vi "main_2CAN.vi"() -> ()   [LabVIEW 2021]
uses:
  <vilib>/xnet/xnet.llb/XNET Frame CAN.ctl
  <vilib>/xnet/xnet.llb/XNET Frame Type CAN.ctl
  Helper functions/General Purpose/measurements.ctl
  Helper functions/General Purpose/measurements_SC.ctl
  Helper functions/Time-sync/time_sync/TypeDef/Synch_shift--cluster.ctl
  <vilib>/Platform/TimedLoop/XDataNode/timing_clust.ctl
  <vilib>/Platform/TimedLoop/XDataNode/nitl_modes.ctl
  <vilib>/Platform/TimedLoop/XDataNode/wakeup.ctl
  Helper functions/communication/PVemulator_Central.ctl
  Helper functions/communication/PVemulator_Central_Info.ctl
  Helper functions/communication/PVemulator_Central_Data.ctl
  Helper functions/communication/SC_references.ctl
  Helper functions/central data acquisition/MeteoBoxCentral.ctl
  Helper functions/central data acquisition/MeteoBoxCentral_Info.ctl
  Helper functions/central data acquisition/MeteoBoxCentral_Data.ctl
  <vilib>/Analysis/baseanly.llb/Mean (DBL).vi
  <vilib>/xnet/xnet.llb/XNET Write (Frame CAN).vi
  <vilib>/xnet/xnet.llb/XNET Read (Frame CAN).vi
  <vilib>/Platform/TimedLoop/XDataNode/XDataNode.xnode
  <vilib>/Platform/TimedLoop/XDataNode/XDNodeRunTimeDep.lvlib
  <userlib>/_OpenG.lib/boolean/boolean.llb/openg_boolean__ogtk.lvlib
  <vilib>/Analysis/NI_AALBase.lvlib
panel:
  out "Finished Late? [i-1]":bool
  out "Iteration Duration":i64
  out "SOC_plot":cluster{"SOC":dbl, "mean":dbl}(graph)
  in  "Vdc_bias":dbl=-4.0 format="%#_13g"
  out "CAN OUT 2":T1 {"payload" format="%x"; "timestamp" format="%<%.7X\n%x>T"; "type" items=["CAN Data"=0, "CAN Remote"=1, "CAN Bus Error"=2, "CAN 2.0 Data"=8, "CAN FD Data"=16, "CAN FD+BRS Data"=24, "J1939 Data"=192, "Delay"=224, "Log Trigger"=225, "Start Trigger"=226]; "identifier" format="%x"}
  out "CAN frame":T1 {"payload" format="%x"; "timestamp" format="%<%.7X\n%x>T"; "type" items=["CAN Data"=0, "CAN Remote"=1, "CAN Bus Error"=2, "CAN 2.0 Data"=8, "CAN FD Data"=16, "CAN FD+BRS Data"=24, "J1939 Data"=192, "Delay"=224, "Log Trigger"=225, "Start Trigger"=226]; "identifier" format="%x"}
  out "Period":i64
  out "time_sc":timestamp
  out "start following SC pre":bool
  out "forming?":bool
  out "Ready SC":bool
  out "OFF SC":bool
  out "V slider 31":dbl(slide) caption="V-i" max=-10.0 scale=0.0..100.0 scale format="%#_4g"
  in  "SEND sp SC":bool
  in  "Start following SC":bool
  in  "Start forming SC":bool
  in  "Vdc SC":dbl=720.0
  out "Synch Monitor":string[][](table)
  in  "Loop Time":u32=125
  out "Error out":errorcluster
  in  "Timeout [ms]":i32=3000
  out "Offset from TR (ns)":dbl
  out "Status Out":T3
  out "ON SC":bool
  out "state SC":u16
  out "measurements SuperCap":T4
  out "V slider 29":dbl(slide) caption="V-i" max=-10.0 scale=650.0..780.0 scale format="%#_4g"
  out "V slider 30":dbl(slide) caption="V-i" max=-10.0 scale=650.0..780.0 scale format="%#_4g"
  out "kW":dbl caption="Numeric" format="%#.3g"
  in  "Pdc SC":dbl
  in  "Shutdwn SC":bool
  in  "Use METEO":bool
  out "Temps":dbl[](array[numeric])
  out "GHIs":dbl[](array[numeric])
  out "Meteo.Tair":dbl
  out "Meteo.GHI":dbl
  in  "Update setpoints":bool
  out "V slider 28":dbl(slide) caption="V-i" max=-10.0 scale=650.0..780.0 scale format="%#_4g"
  out "V slider 27":dbl(slide) caption="V-i" max=-10.0 scale=650.0..780.0 scale format="%#_4g"
  out "V slider 26":dbl(slide) caption="V-i" max=-10.0 scale=650.0..780.0 scale format="%#_4g"
  out "V slider 25":dbl(slide) caption="V-i" max=-10.0 scale=650.0..780.0 scale format="%#_4g"
  out "V slider 24":dbl(slide) caption="V-i" max=-10.0 scale=650.0..780.0 scale format="%#_4g"
  out "V slider 23":dbl(slide) caption="V-i" max=-10.0 scale=650.0..780.0 scale format="%#_4g"
  out "V slider 22":dbl(slide) caption="V-i" max=-10.0 scale=650.0..780.0 scale format="%#_4g"
  out "V slider 21":dbl(slide) caption="V-i" max=-10.0 scale=650.0..780.0 scale format="%#_4g"
  in  "P 4":dbl
  in  "P 3":dbl
  in  "P 2":dbl
  out "state 4":u16
  out "state 3":u16
  out "state 2":u16
  out "state 1":u16
  out "kW":dbl caption="Numeric" format="%#.3g"
  out "kW":dbl caption="Numeric" format="%#.3g"
  out "kW":dbl caption="Numeric" format="%#.3g"
  out "kW":dbl caption="Numeric" format="%#.3g"
  in  "P 1":dbl
  out "current time":timestamp
  in  "measurements":T5
  out "CAN OUT":T1 {"payload" format="%x"; "timestamp" format="%<%.7X\n%x>T"; "type" items=["CAN Data"=0, "CAN Remote"=1, "CAN Bus Error"=2, "CAN 2.0 Data"=8, "CAN FD Data"=16, "CAN FD+BRS Data"=24, "J1939 Data"=192, "Delay"=224, "Log Trigger"=225, "Start Trigger"=226]; "identifier" format="%x"}
  in  "EnablePR 4":bool
  in  "EnablePR 3":bool
  in  "EnablePR 2":bool
  in  "EnablePR 1":bool
  in  "main stop":bool
  in  "DCLinkOK  4":bool
  in  "PowerEnable 4":bool
  in  "ErrAck 4":bool
  in  "Shutdwn 4":bool
  in  "DCLinkOK  3":bool
  in  "PowerEnable 3":bool
  in  "ErrAck 3":bool
  in  "Shutdwn 3":bool
  in  "DCLinkOK 2":bool
  in  "PowerEnable 2":bool
  in  "ErrAck 2":bool
  in  "Shutdwn 2":bool
  out "OFF 4":bool
  out "ON 4":bool
  out "Ready 4":bool
  out "OFF 3":bool
  out "ON 3":bool
  out "Ready 3":bool
  out "OFF 2":bool
  out "ON 2":bool
  out "Ready 2":bool
  out "OFF 1":bool
  out "ON 1":bool
  out "Ready 1":bool
  out "CAN IN":T1 {"payload" format="%x"; "timestamp" format="%<%.7X\n%x>T"; "type" items=["CAN Data"=0, "CAN Remote"=1, "CAN Bus Error"=2, "CAN 2.0 Data"=8, "CAN FD Data"=16, "CAN FD+BRS Data"=24, "J1939 Data"=192, "Delay"=224, "Log Trigger"=225, "Start Trigger"=226]; "identifier" format="%x"}
  in  "CAN [ms]":i64=1
  out "CAN with Conv":bool
  out "Measurements":bool
  in  "Shutdwn 1":bool
  in  "ErrAck 1":bool
  in  "PowerEnable 1":bool
  in  "DCLinkOK 1":bool
  # "PV emulators 1-4"
  # "B22"
  # "DC"
  # "PV 4"
  # "DC"
  # "B21"
  # "DC"
  # "PV 3"
  # "DC"
  # "B20"
  # "DC"
  # "PV 2"
  # "DC"
  # "B19"
  # "1"
  # "DC"
  # "2"
  # "PV 1"
  # "3"
  # "DC"
  # "DC"
  # "SC"
  # "DC"
  # "SOC"
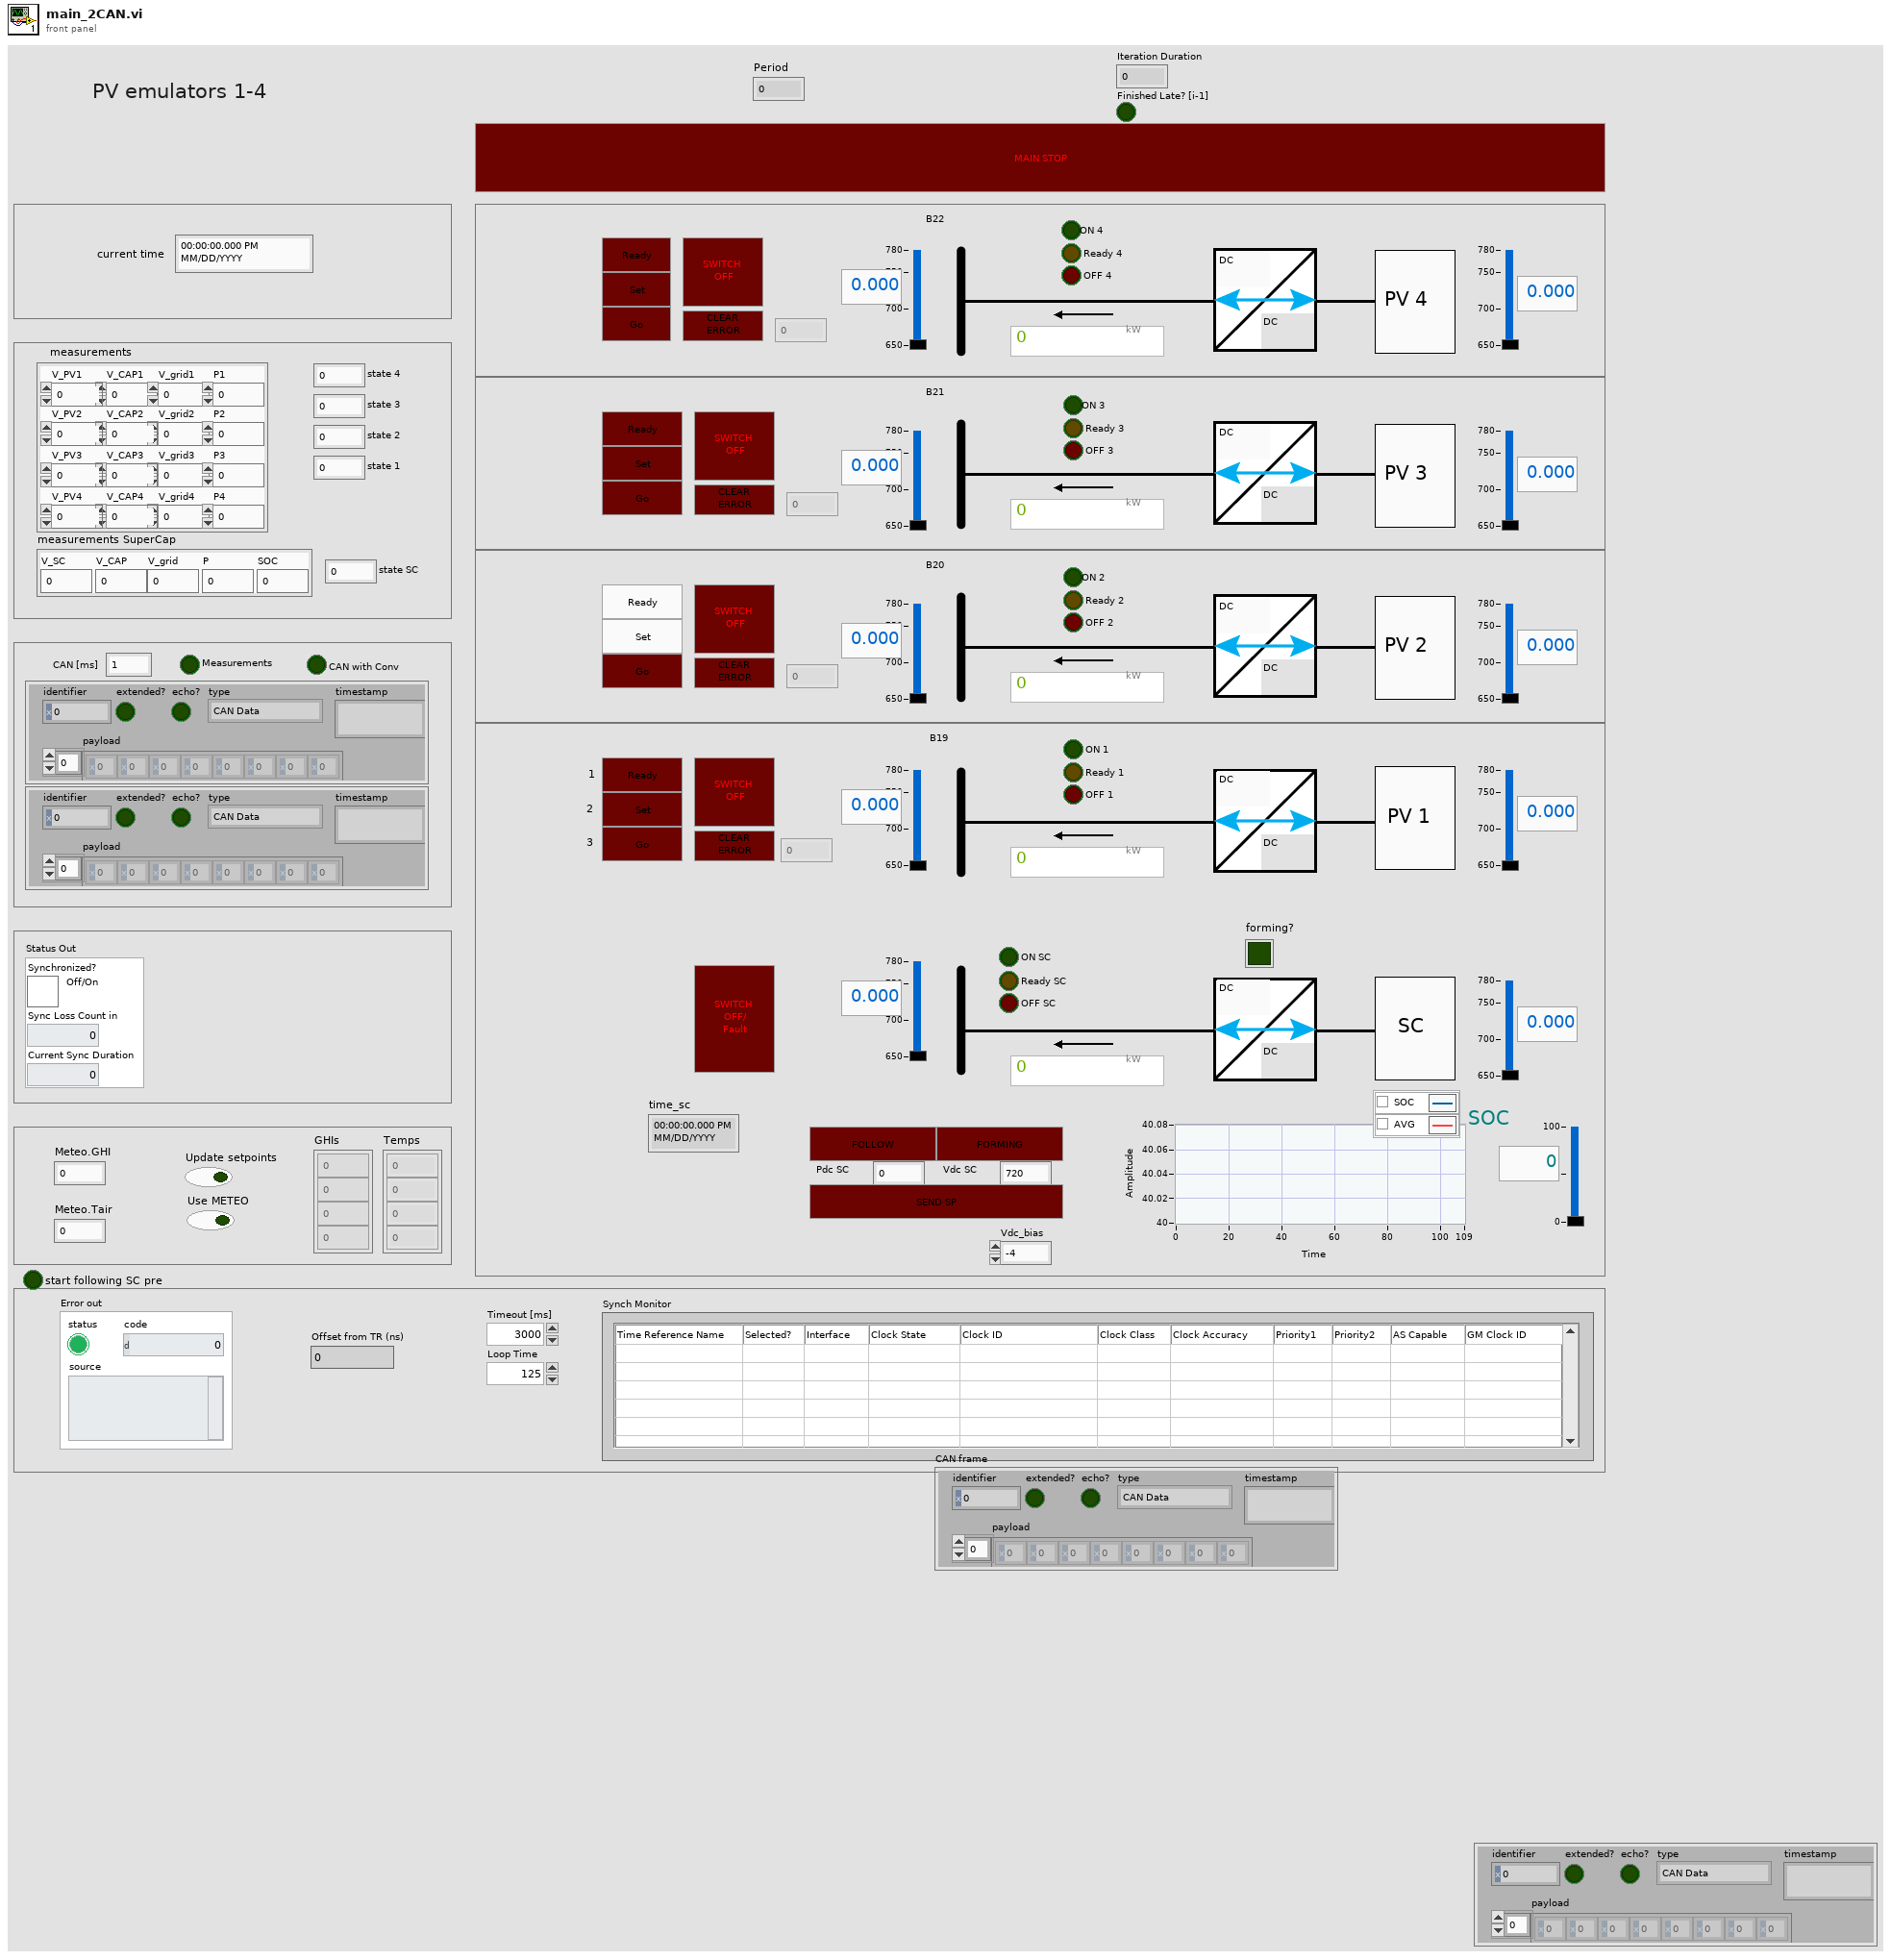
[diagram p1: front panel]
types:
  T1 = typedef "XNET Frame CAN.ctl" = cluster{"timestamp":timestamp, "payload":u8[], "identifier":u32, "type":T2, "extended?":bool, "echo?":bool}
  T2 = typedef "XNET Frame Type CAN.ctl" = u8
  T3 = typedef "Synch_shift--cluster.ctl" = cluster{"Synchronized?":bool, "Sync Loss Count in":u32, "Current Sync Duration":u32}
  T4 = typedef "measurements_SC.ctl" = cluster{"V_SC":dbl, "V_CAP":dbl, "V_grid":dbl, "P":dbl, "SOC":dbl}
  T5 = typedef "measurements.ctl" = cluster{"V_PV1":dbl, "V_CAP1":dbl, "V_PV2":dbl, "V_CAP2":dbl, "V_grid2":dbl, "V_PV3":dbl, "V_CAP3":dbl, "V_grid3":dbl, "V_PV4":dbl, "V_CAP4":dbl, "V_grid4":dbl, "V_grid1":dbl, "P1":dbl, "P2":dbl, "P3":dbl, "P4":dbl}
  T6 = cluster{"Frame In":refnum<k21>, "Frame Out":refnum<k21>}
  T7 = typedef "XDNodeRunTimeDep.lvlib/timing_clust.ctl" = cluster{"Expected End [f-1]":u64, "Actual End [f-1]":u64, "Finished Late? [f-1]":bool, "Expected End [i-1]":u64, "Actual End [i-1]":u64, "Finished Late? [i-1]":bool, "Expected Start [i]":u64, "Actual Start [i]":u64, "Expected Start [f]":u64, "Actual Start [f]":u64, "Source Name":string, "Structure Name":string, "Period":i64, "Deadline":i64, "Offset":i64, "Start":i64, "Priority":i32, "Timeout":i32, "Mode":T8, "Wakeup Reason":T9, "Error":errorcluster, "Source Type":string, "Secondary Source Type":string, "Global End Time":u64, "Global Start Time":u64, "Frame Duration":u64, "Iteration Duration":u64, "Assigned CPU":i32, "I/O Scan Engine Mode":u32}
  T8 = typedef "XDNodeRunTimeDep.lvlib/nitl_modes.ctl" = enum32{"No Change", "Process missed periods, maintain original phase", "Discard missed periods, maintain original phase", "Process missed periods, ignore original phase", "Discard missed periods, ignore original phase"}
  T9 = typedef "XDNodeRunTimeDep.lvlib/wakeup.ctl" = enum32{"Normal", "Aborted", "Asynchronous wakeup", "Timing source error", "Timed loop error", "Timeout"}
  T10 = typedef "MeteoBoxCentral.ctl" = cluster{"Info":T11, "Data":T12}
  T11 = typedef "MeteoBoxCentral_Info.ctl" = cluster{"Resource":string, "Problem":bool, "Timestamp":dbl}
  T12 = typedef "MeteoBoxCentral_Data.ctl" = cluster{"GI":dbl, "GHI":dbl, "GVI":dbl, "Tair":dbl, "Tcell":dbl, "Global_Total_Irr":dbl, "Diffused_Irr":dbl}
  T13 = typedef "PVemulator_Central.ctl" = cluster{"Info":T14, "Data":T15}
  T14 = typedef "PVemulator_Central_Info.ctl" = cluster{"Resource":string, "Problem":bool, "Timestamp":dbl}
  T15 = typedef "PVemulator_Central_Data.ctl" = cluster{"Status 1":bool, "Status 2":bool, "measurements":T5, "Status 3":bool, "Status 4":bool, "measurements SC":T4, "Status SC":bool, "Forming/Following":bool, "Start forming":bool, "SC references":T16, "Start following":bool}
  T16 = typedef "SC_references.ctl" = cluster{"Vdc":dbl, "Pdc":dbl}
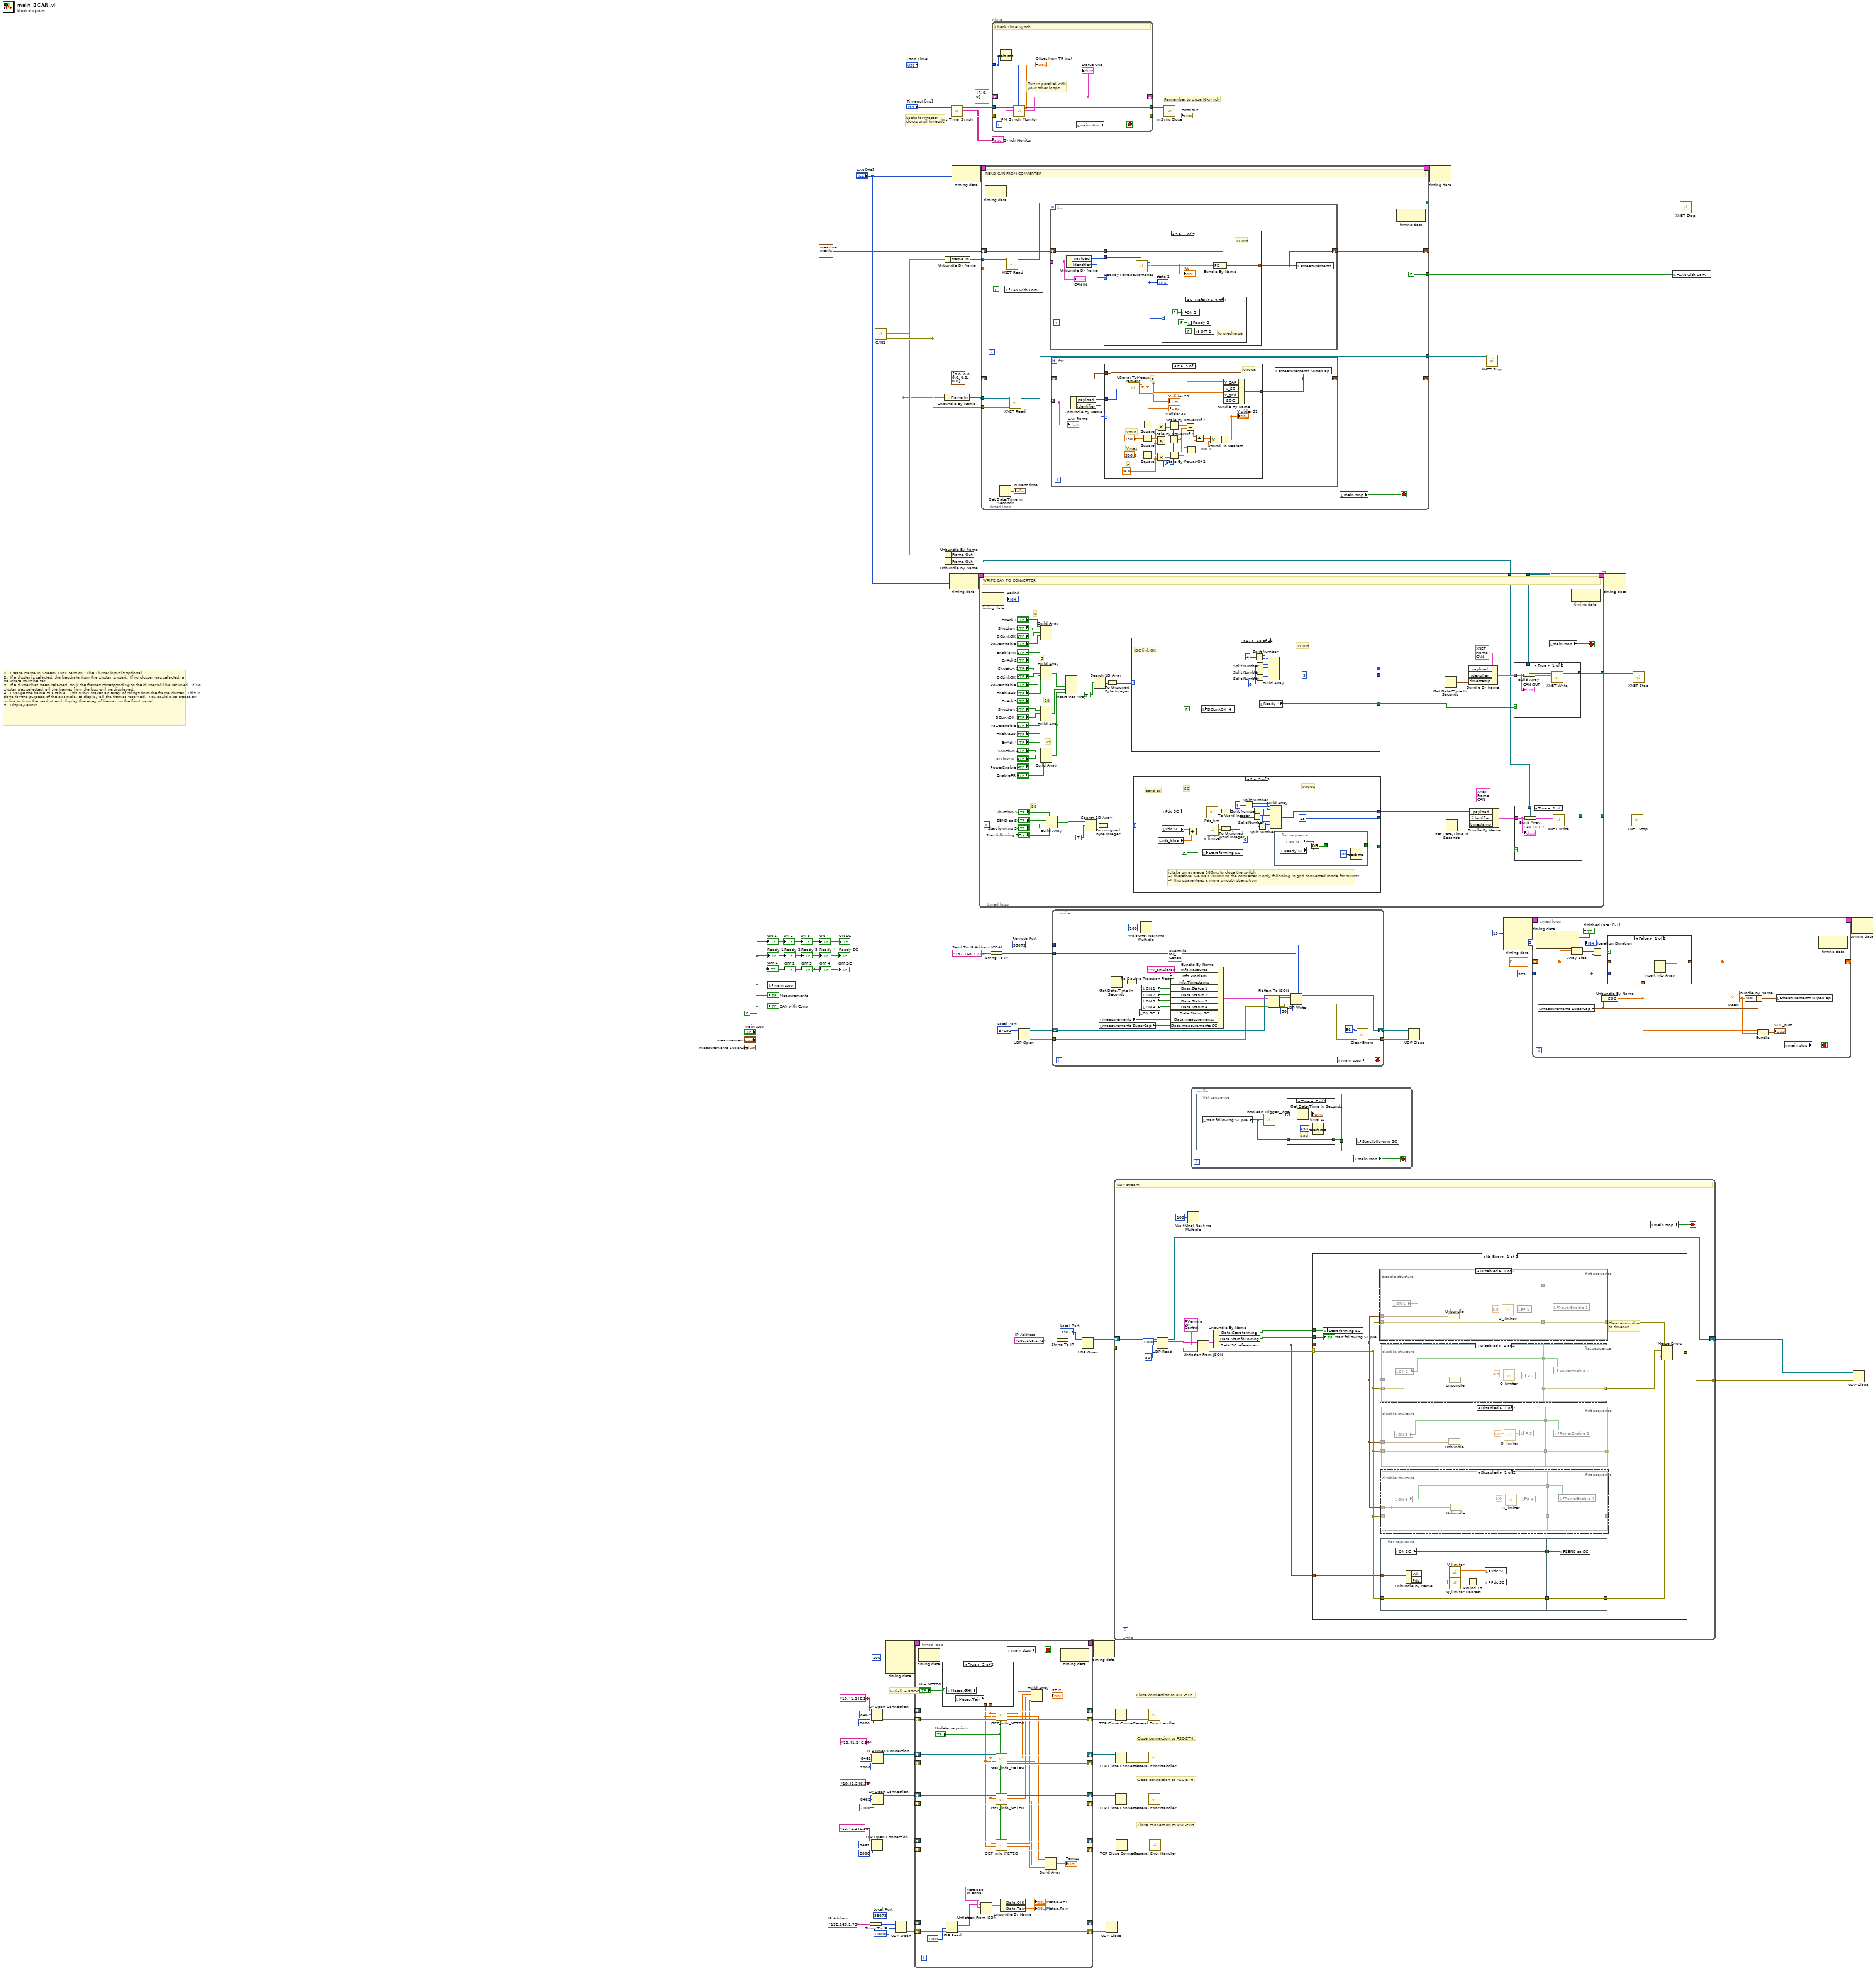
[diagram p0: block diagram]
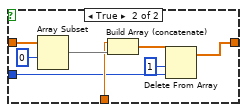
[diagram p2: hidden frame]
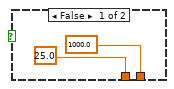
[diagram p9: hidden frame]
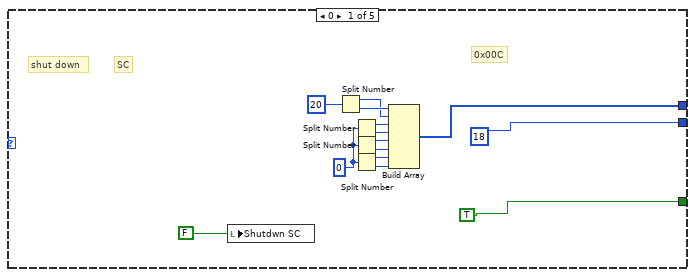
[diagram p11: hidden frame]
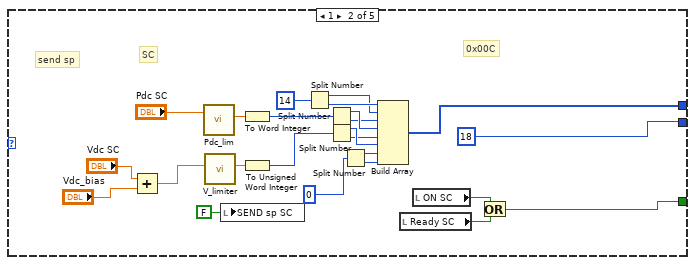
[diagram p12: hidden frame]
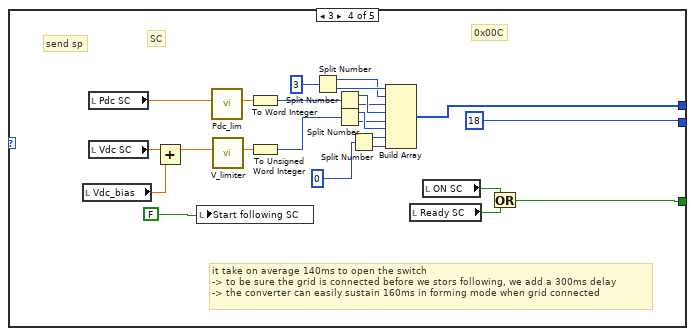
[diagram p13: hidden frame]
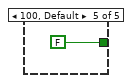
[diagram p14: hidden frame]
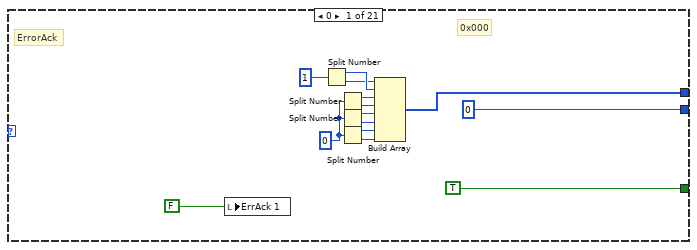
[diagram p16: hidden frame]
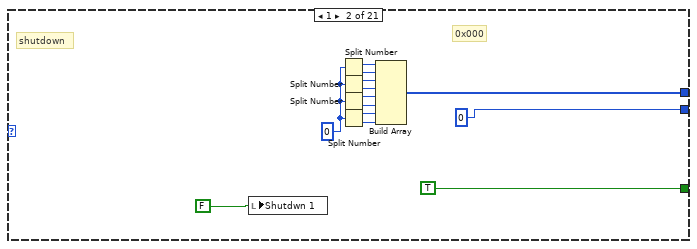
[diagram p17: hidden frame]
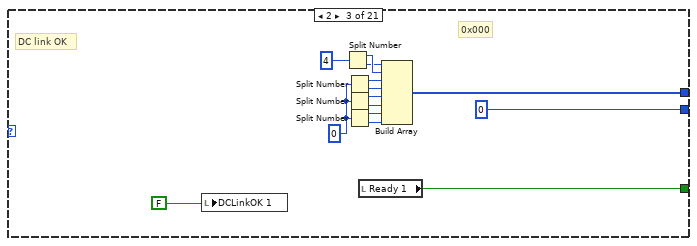
[diagram p18: hidden frame]
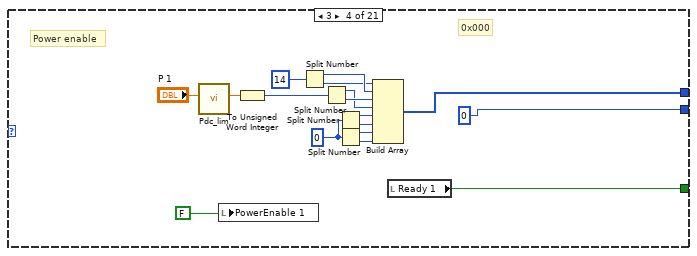
[diagram p19: hidden frame]
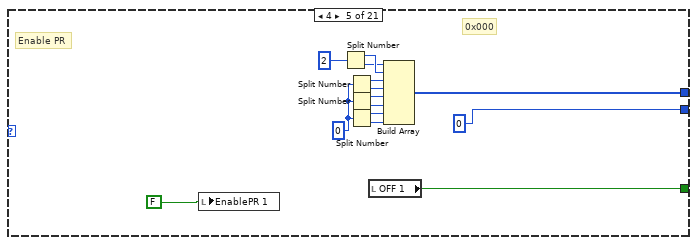
[diagram p20: hidden frame]
diagram:
  w28 = u16 33073  # Local Port
  w29 = "192.168.1.73"  # IP Address
  w69 = u16 39073  # Local Port
  w70 = "192.168.1.73"  # IP Address
  w84 = u16 37692  # Local Port
  w22 = u16 35073  # Remote Port
  w83 = "192.168.1.210"  # Send To IP Address (CDA)
  w16 = FALSE
  # "Remember to close NI-synch"
  # "Looks for master \nclocks until timeout"
  # "Close connection to PSC-ETH."
  # "Close connection to PSC-ETH."
  # "Close connection to PSC-ETH."
  # "Close connection to PSC-ETH."
  # "Initialize PSC-ETH"
  # "1.  Create Frame In Stream XNET session.  The Cluster input is optional.  \n2.  If a cluster is selected, the baudrate from the cluster is used.  If no cluster was selected, a baudrate must be set.\n3.  If a cluster has been selected, only the frames corresponding to the cluster will be returned.  If no cluster was selected, all the frames from the bus will be displayed.\n4.  Change the frame to a table.  This subVI makes an array of strings from the frame cluster.  This is done for the purpose of the example, to display all the frames received.  You could also create an indicator from the read VI and display the array of frames on the front panel. \n5.  Display errors."
  n1 = local write "main stop"(w16) -> ()
  n2 = String To IP(1:w70) -> (0:w71:u32)
  n3 = TCP Open Connection(address="10.41.246.39", remote port or service name=u16 8462 ("remote port"), timeout ms (60000)=2000) -> (connection ID=w54:refnum<k5>, error out=w53:errorcluster)  [unwired: 2 in]
  n4 = TCP Open Connection(address="10.41.246.36", remote port or service name=u16 8462 ("remote port"), timeout ms (60000)=2000) -> (connection ID=w76:refnum<k5>, error out=w75:errorcluster)  [unwired: 2 in]
  n5 = TCP Open Connection(address="10.41.246.38", remote port or service name=u16 8462 ("remote port"), timeout ms (60000)=2000) -> (connection ID=w56:refnum<k5>, error out=w55:errorcluster)  [unwired: 2 in]
  n6 = TCP Open Connection(address="10.41.246.37", remote port or service name=u16 8462 ("remote port"), timeout ms (60000)=2000) -> (connection ID=w58:refnum<k5>, error out=w57:errorcluster)  [unwired: 2 in]
  n7 = call "CAN2.vi"() -> ("error out"=w12:errorcluster, "CAN 2"=w8:T6, "CAN1"=w9:T6)  [unwired: 8 in, 1 out]
  n8 = node-c288(i64 100 ("Period")) -> (w82:T7)  [unwired: 3 in]
  n9 = UDP Open(7:w71, 9:10000 ("timeout ms (25000)"), 11:w69) -> (port=w43:refnum<k16>, 0:w42:errorcluster)  [unwired: 2 in, 1 out]
  n10 = timed-loop {
    timing: w82 -> [_]
    timing-out: [_] -> w81
    shift-right: [w130] -> w73
    shift-left: w76 -> [w132]
    shift-right: [w129] -> w72
    shift-left: w75 -> [w131]
    shift-right: [w121] -> w48
    shift-left: w57 -> [w127]
    shift-right: [w122] -> w49
    shift-left: w58 -> [w128]
    shift-right: [w120] -> w47
    shift-left: w56 -> [w126]
    shift-right: [w119] -> w46
    shift-left: w55 -> [w125]
    shift-right: [w118] -> w45
    shift-left: w54 -> [w124]
    shift-right: [w117] -> w44
    shift-left: w53 -> [w123]
    shift-right: [w95] -> w41
    shift-left: w43 -> [w97]
    shift-right: [w94] -> w40
    shift-left: w42 -> [w96]
    stop <- w133 stop-if-true
    n11 = node-c288() -> ()  [unwired: 1 in, 1 out]
    n12 = case shown="True" "Use METEO" {
      tunnel: [1000.0 ("Meteo.GHI") w136] -> w115
      tunnel: [25.0 ("Meteo.Tair") w137] -> w114
      frame False {
      }
      frame True {
        n13 = local read "Meteo.GHI"() -> (w136:dbl)
        n14 = local read "Meteo.Tair"() -> (w137:dbl)
      }
    }
    n15 = UDP Read(connection ID=w97, timeout ms (25000)=1000, 8:w96) -> (data out=w99:string, error out=w94:errorcluster, 3:w95:refnum<k16>)  [unwired: 1 in, 2 out]
    n16 = Unflatten From JSON(JSON string=w99, type and defaults=T10 {"Info"={"Resource"="MeteoBox", "Problem"=FALSE, "Timestamp"=0.0}, "Data"={"GI"=0.0, "GHI"=0.0, "GVI"=0.0, "Tair"=0.0, "Tcell"=0.0, "Global_Total_Irr"=0.0, "Diffused_Irr"=0.0}} ("Cluster")) -> (value=w101:T10)  [unwired: 5 in, 1 out]
    n17 = call "GET_info_METEO.vi"("Update GHI"="Update setpoints", "error in"=w131, "set Temp"=w114, "set GHI"=w115, "connection ID in"=w132) -> ("error out"=w129:errorcluster, "read Temp"=w105:dbl, "read GHI"=w113:dbl, "connection ID out"=w130:refnum<k5>)  [unwired: 3 in]
    n18 = call "GET_info_METEO.vi"("Update GHI"="Update setpoints", "error in"=w127, "set Temp"=w114, "set GHI"=w115, "connection ID in"=w128) -> ("error out"=w121:errorcluster, "read Temp"=w106:dbl, "read GHI"=w112:dbl, "connection ID out"=w122:refnum<k5>)  [unwired: 3 in]
    n19 = call "GET_info_METEO.vi"("Update GHI"="Update setpoints", "error in"=w125, "set Temp"=w114, "set GHI"=w115, "connection ID in"=w126) -> ("error out"=w119:errorcluster, "read Temp"=w107:dbl, "read GHI"=w111:dbl, "connection ID out"=w120:refnum<k5>)  [unwired: 3 in]
    n20 = call "GET_info_METEO.vi"("Update GHI"="Update setpoints", "error in"=w123, "set Temp"=w114, "set GHI"=w115, "connection ID in"=w124) -> ("error out"=w117:errorcluster, "read Temp"=w108:dbl, "read GHI"=w110:dbl, "connection ID out"=w118:refnum<k5>)  [unwired: 3 in]
    n21 = Unbundle By Name(w101) -> ("Data.GHI"=→"Meteo.GHI":dbl, "Data.Tair"=→"Meteo.Tair":dbl)
    n22 = local read "main stop"() -> (w133:bool)
    n23 = Build Array(w113, w112, w111, w110) -> (→"GHIs":dbl[])
    n24 = Build Array(w105, w106, w107, w108) -> (→"Temps":dbl[])
    n25 = node-c288() -> ()  [unwired: 1 in, 1 out]
  }
  n26 = Unbundle By Name(w8) -> ("Frame In"=w10:refnum<k21>)
  n27 = Unbundle By Name(w9) -> ("Frame In"=w11:refnum<k21>)
  n28 = Unbundle By Name(w9) -> ("Frame Out"=w6:refnum<k21>)
  n29 = Unbundle By Name(w8) -> ("Frame Out"=w7:refnum<k21>)
  n30 = node-c288("CAN [ms]") -> (w86:T7)
  n31 = call "Init_Time_Synch.vi"("Timeout [ms]"="Timeout [ms]") -> ("Error out"=w38:errorcluster, "Synch Monitor"=→"Synch Monitor":string[][], "Synch Out"=w36:refnum<k15>)  [unwired: 7 in, 1 out]
  n32 = node-c288("CAN [ms]") -> (w89:T7)
  n33 = timed-loop {
    tunnel: w6 -> [w189]
    tunnel: [w188] -> w91
    timing: w86 -> [_]
    timing-out: [_] -> w85
    tunnel: [w144] -> w13
    tunnel: w7 -> [w140]
    stop <- w187 stop-if-true
    # "15"
    # "10"
    # "5"
    # "0"
    # "20"
    # "WRITE CAN TO CONVERTER"
    n34 = node-c288() -> (→"Period":i64)  [unwired: 1 in]
    n35 = Build Array("ErrAck 1", "Shutdwn 1", "DCLinkOK 1", "PowerEnable 1", "EnablePR 1") -> (w168:bool[])
    n36 = Build Array("ErrAck 2", "Shutdwn 2", "DCLinkOK 2", "PowerEnable 2", "EnablePR 2") -> (w167:bool[])
    n37 = Build Array("ErrAck 3", "Shutdwn 3", "DCLinkOK  3", "PowerEnable 3", "EnablePR 3") -> (w166:bool[])
    n38 = Build Array("ErrAck 4", "Shutdwn 4", "DCLinkOK  4", "PowerEnable 4", "EnablePR 4") -> (w165:bool[])
    n39 = Build Array("Shutdwn SC", "SEND sp SC", "Start forming SC", "Start following SC") -> (w149:bool[])
    n40 = Insert Into Array(array=w168, new element #1=w167, new element #2=w166, new element #3=w165) -> (w164:bool[])  [unwired: 1 in]
    n41 = Search 1D Array(1D array=w149, element=TRUE) -> (index of element=w150:i32)  [unwired: 1 in]
    n42 = Search 1D Array(1D array=w164, element=TRUE) -> (index of element=w183:i32)  [unwired: 1 in]
    n43 = To Unsigned Byte Integer(number=w150) -> (unsigned 8bit integer=w148:u8)
    n44 = To Unsigned Byte Integer(number=w183) -> (unsigned 8bit integer=w159:u8)
    n45 = case shown="17" w159 {
      tunnel: [u32 0 ("identifier") u32 0 ("identifier") u32 0 ("identifier") u32 0 ("identifier") u32 0 ("identifier") u32 3 ("identifier") u32 3 ("identifier") u32 3 ("identifier") u32 3 ("identifier") u32 3 ("identifier") u32 6 ("identifier") u32 6 ("identifier") u32 6 ("identifier") u32 6 ("identifier") u32 6 ("identifier") u32 9 ("identifier") u32 9 ("identifier") u32 9 ("identifier") u32 9 ("identifier") u32 9 ("identifier") _] -> w193
      tunnel: [TRUE TRUE w323 w337 w354 TRUE TRUE w395 w409 w426 TRUE TRUE w467 w481 w498 TRUE TRUE w539 w553 w570 FALSE] -> w191
      tunnel: [w299 w311 w328 w344 w358 w371 w383 w400 w416 w430 w443 w455 w472 w488 w502 w515 w527 w544 w560 w574 _] -> w158
      frame 0 {
        w300 = u16 0 ("element")
        # "0x000"
        # "ErrorAck"
        n46 = local write "ErrAck 1"(FALSE ("SEND sp")) -> ()
        n47 = Split Number(x=u16 1) -> (hi(x)=w297:u8, lo(x)=w296:u8)
        n48 = Split Number(x=w300) -> (hi(x)=w306:u8, lo(x)=w305:u8)
        n49 = Split Number(x=w300) -> (hi(x)=w304:u8, lo(x)=w303:u8)
        n50 = Split Number(x=w300) -> (hi(x)=w302:u8, lo(x)=w301:u8)
        n51 = Build Array(w296, w297, w306, w305, w304, w303, w302, w301) -> (w299:u8[])
      }
      frame 1 {
        w310 = u16 0 ("element")
        # "0x000"
        # "shutdown"
        n52 = local write "Shutdwn 1"(FALSE ("SEND sp")) -> ()
        n53 = Split Number(x=w310) -> (hi(x)=w319:u8, lo(x)=w318:u8)
        n54 = Split Number(x=w310) -> (hi(x)=w317:u8, lo(x)=w316:u8)
        n55 = Split Number(x=w310) -> (hi(x)=w315:u8, lo(x)=w314:u8)
        n56 = Split Number(x=w310) -> (hi(x)=w313:u8, lo(x)=w312:u8)
        n57 = Build Array(w319, w318, w317, w316, w315, w314, w313, w312) -> (w311:u8[])
      }
      frame 2 {
        w329 = u16 0 ("element")
        # "0x000"
        # "DC link OK"
        n58 = local write "DCLinkOK 1"(FALSE ("SEND sp")) -> ()
        n59 = Split Number(x=u16 4) -> (hi(x)=w325:u8, lo(x)=w324:u8)
        n60 = Split Number(x=w329) -> (hi(x)=w335:u8, lo(x)=w334:u8)
        n61 = Split Number(x=w329) -> (hi(x)=w333:u8, lo(x)=w332:u8)
        n62 = Split Number(x=w329) -> (hi(x)=w331:u8, lo(x)=w330:u8)
        n63 = local read "Ready 1"() -> (w323:bool)
        n64 = Build Array(w324, w325, w335, w334, w333, w332, w331, w330) -> (w328:u8[])
      }
      frame 3 {
        w345 = u16 0 ("element")
        # "0x000"
        # "Power enable"
        n65 = call "Pdc_lim.vi"("IN Vdc"="P 1") -> ("OUT Vdc"=w350:dbl)  [unwired: 10 in]
        n66 = local write "PowerEnable 1"(FALSE ("SEND sp")) -> ()
        n67 = To Unsigned Word Integer(number=w350) -> (unsigned 16bit integer=w343:u16)
        n68 = Split Number(x=u16 14) -> (hi(x)=w341:u8, lo(x)=w340:u8)
        n69 = Split Number(x=w343) -> (hi(x)=w338:u8, lo(x)=w339:u8)
        n70 = Split Number(x=w345) -> (hi(x)=w349:u8, lo(x)=w348:u8)
        n71 = Split Number(x=w345) -> (hi(x)=w347:u8, lo(x)=w346:u8)
        n72 = Build Array(w340, w341, w339, w338, w349, w348, w347, w346) -> (w344:u8[])
        n73 = local read "Ready 1"() -> (w337:bool)
      }
      frame 4 {
        w359 = u16 0 ("element")
        # "0x000"
        # "Enable PR"
        n74 = local write "EnablePR 1"(FALSE ("SEND sp")) -> ()
        n75 = Split Number(x=u16 2) -> (hi(x)=w356:u8, lo(x)=w355:u8)
        n76 = Split Number(x=w359) -> (hi(x)=w365:u8, lo(x)=w364:u8)
        n77 = Split Number(x=w359) -> (hi(x)=w363:u8, lo(x)=w362:u8)
        n78 = Split Number(x=w359) -> (hi(x)=w361:u8, lo(x)=w360:u8)
        n79 = local read "OFF 1"() -> (w354:bool)
        n80 = Build Array(w355, w356, w365, w364, w363, w362, w361, w360) -> (w358:u8[])
      }
      frame 5 {
        w372 = u16 0 ("element")
        # "0x003"
        # "ErrorAck"
        n81 = local write "ErrAck 2"(FALSE ("SEND sp")) -> ()
        n82 = Split Number(x=u16 1) -> (hi(x)=w369:u8, lo(x)=w368:u8)
        n83 = Split Number(x=w372) -> (hi(x)=w378:u8, lo(x)=w377:u8)
        n84 = Split Number(x=w372) -> (hi(x)=w376:u8, lo(x)=w375:u8)
        n85 = Split Number(x=w372) -> (hi(x)=w374:u8, lo(x)=w373:u8)
        n86 = Build Array(w368, w369, w378, w377, w376, w375, w374, w373) -> (w371:u8[])
      }
      frame 6 {
        w382 = u16 0 ("element")
        # "0x003"
        # "shutdown"
        n87 = local write "Shutdwn 2"(FALSE ("SEND sp")) -> ()
        n88 = Split Number(x=w382) -> (hi(x)=w391:u8, lo(x)=w390:u8)
        n89 = Split Number(x=w382) -> (hi(x)=w389:u8, lo(x)=w388:u8)
        n90 = Split Number(x=w382) -> (hi(x)=w387:u8, lo(x)=w386:u8)
        n91 = Split Number(x=w382) -> (hi(x)=w385:u8, lo(x)=w384:u8)
        n92 = Build Array(w391, w390, w389, w388, w387, w386, w385, w384) -> (w383:u8[])
      }
      frame 7 {
        w401 = u16 0 ("element")
        # "0x003"
        # "DC link OK"
        n93 = local write "DCLinkOK 2"(FALSE ("SEND sp")) -> ()
        n94 = Split Number(x=u16 4) -> (hi(x)=w397:u8, lo(x)=w396:u8)
        n95 = Split Number(x=w401) -> (hi(x)=w407:u8, lo(x)=w406:u8)
        n96 = Split Number(x=w401) -> (hi(x)=w405:u8, lo(x)=w404:u8)
        n97 = Split Number(x=w401) -> (hi(x)=w403:u8, lo(x)=w402:u8)
        n98 = local read "Ready 2"() -> (w395:bool)
        n99 = Build Array(w396, w397, w407, w406, w405, w404, w403, w402) -> (w400:u8[])
      }
      frame 8 {
        w417 = u16 0 ("element")
        # "0x003"
        # "Power enable"
        n100 = call "Pdc_lim.vi"("IN Vdc"="P 2") -> ("OUT Vdc"=w422:dbl)  [unwired: 10 in]
        n101 = local write "PowerEnable 2"(FALSE ("SEND sp")) -> ()
        n102 = To Unsigned Word Integer(number=w422) -> (unsigned 16bit integer=w415:u16)
        n103 = Split Number(x=u16 14) -> (hi(x)=w413:u8, lo(x)=w412:u8)
        n104 = Split Number(x=w415) -> (hi(x)=w410:u8, lo(x)=w411:u8)
        n105 = Split Number(x=w417) -> (hi(x)=w421:u8, lo(x)=w420:u8)
        n106 = Split Number(x=w417) -> (hi(x)=w419:u8, lo(x)=w418:u8)
        n107 = Build Array(w412, w413, w411, w410, w421, w420, w419, w418) -> (w416:u8[])
        n108 = local read "Ready 2"() -> (w409:bool)
      }
      frame 9 {
        w431 = u16 0 ("element")
        # "0x003"
        # "Enable PR"
        n109 = local write "EnablePR 2"(FALSE ("SEND sp")) -> ()
        n110 = Split Number(x=u16 2) -> (hi(x)=w428:u8, lo(x)=w427:u8)
        n111 = Split Number(x=w431) -> (hi(x)=w437:u8, lo(x)=w436:u8)
        n112 = Split Number(x=w431) -> (hi(x)=w435:u8, lo(x)=w434:u8)
        n113 = Split Number(x=w431) -> (hi(x)=w433:u8, lo(x)=w432:u8)
        n114 = local read "OFF 2"() -> (w426:bool)
        n115 = Build Array(w427, w428, w437, w436, w435, w434, w433, w432) -> (w430:u8[])
      }
      frame 10 {
        w444 = u16 0 ("element")
        # "0x006"
        # "ErrorAck"
        n116 = local write "ErrAck 3"(FALSE ("SEND sp")) -> ()
        n117 = Split Number(x=u16 1) -> (hi(x)=w441:u8, lo(x)=w440:u8)
        n118 = Split Number(x=w444) -> (hi(x)=w450:u8, lo(x)=w449:u8)
        n119 = Split Number(x=w444) -> (hi(x)=w448:u8, lo(x)=w447:u8)
        n120 = Split Number(x=w444) -> (hi(x)=w446:u8, lo(x)=w445:u8)
        n121 = Build Array(w440, w441, w450, w449, w448, w447, w446, w445) -> (w443:u8[])
      }
      frame 11 {
        w454 = u16 0 ("element")
        # "0x006"
        # "shutdown"
        n122 = local write "Shutdwn 3"(FALSE ("SEND sp")) -> ()
        n123 = Split Number(x=w454) -> (hi(x)=w463:u8, lo(x)=w462:u8)
        n124 = Split Number(x=w454) -> (hi(x)=w461:u8, lo(x)=w460:u8)
        n125 = Split Number(x=w454) -> (hi(x)=w459:u8, lo(x)=w458:u8)
        n126 = Split Number(x=w454) -> (hi(x)=w457:u8, lo(x)=w456:u8)
        n127 = Build Array(w463, w462, w461, w460, w459, w458, w457, w456) -> (w455:u8[])
      }
      frame 12 {
        w473 = u16 0 ("element")
        # "0x006"
        # "DC link OK"
        n128 = local write "DCLinkOK  3"(FALSE ("SEND sp")) -> ()
        n129 = Split Number(x=u16 4) -> (hi(x)=w469:u8, lo(x)=w468:u8)
        n130 = Split Number(x=w473) -> (hi(x)=w479:u8, lo(x)=w478:u8)
        n131 = Split Number(x=w473) -> (hi(x)=w477:u8, lo(x)=w476:u8)
        n132 = Split Number(x=w473) -> (hi(x)=w475:u8, lo(x)=w474:u8)
        n133 = local read "Ready 3"() -> (w467:bool)
        n134 = Build Array(w468, w469, w479, w478, w477, w476, w475, w474) -> (w472:u8[])
      }
      frame 13 {
        w489 = u16 0 ("element")
        # "0x006"
        # "Power enable"
        n135 = call "Pdc_lim.vi"("IN Vdc"="P 3") -> ("OUT Vdc"=w494:dbl)  [unwired: 10 in]
        n136 = local write "PowerEnable 3"(FALSE ("SEND sp")) -> ()
        n137 = To Unsigned Word Integer(number=w494) -> (unsigned 16bit integer=w487:u16)
        n138 = Split Number(x=u16 14) -> (hi(x)=w485:u8, lo(x)=w484:u8)
        n139 = Split Number(x=w487) -> (hi(x)=w482:u8, lo(x)=w483:u8)
        n140 = Split Number(x=w489) -> (hi(x)=w493:u8, lo(x)=w492:u8)
        n141 = Split Number(x=w489) -> (hi(x)=w491:u8, lo(x)=w490:u8)
        n142 = Build Array(w484, w485, w483, w482, w493, w492, w491, w490) -> (w488:u8[])
        n143 = local read "Ready 3"() -> (w481:bool)
      }
      frame 14 {
        w503 = u16 0 ("element")
        # "0x006"
        # "Enable PR"
        n144 = local write "EnablePR 3"(FALSE ("SEND sp")) -> ()
        n145 = Split Number(x=u16 2) -> (hi(x)=w500:u8, lo(x)=w499:u8)
        n146 = Split Number(x=w503) -> (hi(x)=w509:u8, lo(x)=w508:u8)
        n147 = Split Number(x=w503) -> (hi(x)=w507:u8, lo(x)=w506:u8)
        n148 = Split Number(x=w503) -> (hi(x)=w505:u8, lo(x)=w504:u8)
        n149 = local read "OFF 3"() -> (w498:bool)
        n150 = Build Array(w499, w500, w509, w508, w507, w506, w505, w504) -> (w502:u8[])
      }
      frame 15 {
        w516 = u16 0 ("element")
        # "0x009"
        # "ErrorAck"
        n151 = local write "ErrAck 4"(FALSE ("SEND sp")) -> ()
        n152 = Split Number(x=u16 1) -> (hi(x)=w513:u8, lo(x)=w512:u8)
        n153 = Split Number(x=w516) -> (hi(x)=w522:u8, lo(x)=w521:u8)
        n154 = Split Number(x=w516) -> (hi(x)=w520:u8, lo(x)=w519:u8)
        n155 = Split Number(x=w516) -> (hi(x)=w518:u8, lo(x)=w517:u8)
        n156 = Build Array(w512, w513, w522, w521, w520, w519, w518, w517) -> (w515:u8[])
      }
      frame 16 {
        w526 = u16 0 ("element")
        # "0x009"
        # "shutdown"
        n157 = local write "Shutdwn 4"(FALSE ("SEND sp")) -> ()
        n158 = Split Number(x=w526) -> (hi(x)=w535:u8, lo(x)=w534:u8)
        n159 = Split Number(x=w526) -> (hi(x)=w533:u8, lo(x)=w532:u8)
        n160 = Split Number(x=w526) -> (hi(x)=w531:u8, lo(x)=w530:u8)
        n161 = Split Number(x=w526) -> (hi(x)=w529:u8, lo(x)=w528:u8)
        n162 = Build Array(w535, w534, w533, w532, w531, w530, w529, w528) -> (w527:u8[])
      }
      frame 17 {
        w545 = u16 0 ("element")
        # "0x009"
        # "DC link OK"
        n163 = local write "DCLinkOK  4"(FALSE ("SEND sp")) -> ()
        n164 = Split Number(x=u16 4) -> (hi(x)=w541:u8, lo(x)=w540:u8)
        n165 = Split Number(x=w545) -> (hi(x)=w551:u8, lo(x)=w550:u8)
        n166 = Split Number(x=w545) -> (hi(x)=w549:u8, lo(x)=w548:u8)
        n167 = Split Number(x=w545) -> (hi(x)=w547:u8, lo(x)=w546:u8)
        n168 = local read "Ready 4"() -> (w539:bool)
        n169 = Build Array(w540, w541, w551, w550, w549, w548, w547, w546) -> (w544:u8[])
      }
      frame 18 {
        w561 = u16 0 ("element")
        # "0x009"
        # "Power enable"
        n170 = call "Pdc_lim.vi"("IN Vdc"="P 4") -> ("OUT Vdc"=w566:dbl)  [unwired: 10 in]
        n171 = local write "PowerEnable 4"(FALSE ("SEND sp")) -> ()
        n172 = To Unsigned Word Integer(number=w566) -> (unsigned 16bit integer=w559:u16)
        n173 = Split Number(x=u16 14) -> (hi(x)=w557:u8, lo(x)=w556:u8)
        n174 = Split Number(x=w559) -> (hi(x)=w554:u8, lo(x)=w555:u8)
        n175 = Split Number(x=w561) -> (hi(x)=w565:u8, lo(x)=w564:u8)
        n176 = Split Number(x=w561) -> (hi(x)=w563:u8, lo(x)=w562:u8)
        n177 = Build Array(w556, w557, w555, w554, w565, w564, w563, w562) -> (w560:u8[])
        n178 = local read "Ready 4"() -> (w553:bool)
      }
      frame 19 {
        w575 = u16 0 ("element")
        # "0x009"
        # "Enable PR"
        n179 = local write "EnablePR 4"(FALSE ("SEND sp")) -> ()
        n180 = Split Number(x=u16 2) -> (hi(x)=w572:u8, lo(x)=w571:u8)
        n181 = Split Number(x=w575) -> (hi(x)=w581:u8, lo(x)=w580:u8)
        n182 = Split Number(x=w575) -> (hi(x)=w579:u8, lo(x)=w578:u8)
        n183 = Split Number(x=w575) -> (hi(x)=w577:u8, lo(x)=w576:u8)
        n184 = local read "OFF 4"() -> (w570:bool)
        n185 = Build Array(w571, w572, w581, w580, w579, w578, w577, w576) -> (w574:u8[])
      }
      frame 100, Default {
      }
    }
    n186 = case shown="2" w148 {
      tunnel: [w200 w217 w240 w266 _] -> w143
      tunnel: [u32 18 ("identifier") u32 18 ("identifier") u32 18 ("identifier") u32 18 ("identifier") _] -> w142
      tunnel: [TRUE w215 w238 w268 FALSE] -> w141
      frame 0 {
        w208 = u16 0 ("element")
        # "SC"
        # "0x00C"
        # "shut down"
        n187 = local write "Shutdwn SC"(FALSE ("SEND sp")) -> ()
        n188 = Split Number(x=u16 20) -> (hi(x)=w210:u8, lo(x)=w211:u8)
        n189 = Split Number(x=w208) -> (hi(x)=w202:u8, lo(x)=w203:u8)
        n190 = Split Number(x=w208) -> (hi(x)=w204:u8, lo(x)=w205:u8)
        n191 = Split Number(x=w208) -> (hi(x)=w206:u8, lo(x)=w207:u8)
        n192 = Build Array(w211, w210, w202, w203, w204, w205, w206, w207) -> (w200:u8[])
      }
      frame 1 {
        # "SC"
        # "0x00C"
        # "send sp"
        n193 = Add(x="Vdc SC", y="Vdc_bias") -> (x+y=w213:dbl)
        n194 = call "Pdc_lim.vi"("IN Vdc"="Pdc SC") -> ("OUT Vdc"=w218:dbl)  [unwired: 10 in]
        n195 = call "V_limiter.vi"("IN Q"=w213) -> ("OUT Q"=w229:dbl)  [unwired: 10 in]
        n196 = local write "SEND sp SC"(FALSE ("SEND sp SC")) -> ()
        n197 = To Word Integer(number=w218) -> (16bit integer=w222:i16)
        n198 = To Unsigned Word Integer(number=w229) -> (unsigned 16bit integer=w230:u16)
        n199 = Split Number(x=u16 14) -> (hi(x)=w224:u8, lo(x)=w225:u8)
        n200 = Split Number(x=w222) -> (hi(x)=w227:u8, lo(x)=w226:u8)
        n201 = Split Number(x=w230) -> (hi(x)=w232:u8, lo(x)=w231:u8)
        n202 = Split Number(x=u16 0 ("element")) -> (hi(x)=w219:u8, lo(x)=w220:u8)
        n203 = Build Array(w225, w224, w226, w227, w231, w232, w219, w220) -> (w217:u8[])
        n204 = local read "Ready SC"() -> (w235:bool)
        n205 = local read "ON SC"() -> (w234:bool)
        n206 = Or(x=w234, y=w235) -> (x .or. y?=w215:bool)
      }
      frame 2 {
        # "it take on average 500ms to close the switch\n-> therefore, we wait 200ms so the converter is only following in grid connected mode for 300ms\n-> this guarentees a more smooth stransition"
        # "SC"
        # "0x00C"
        # "send sp"
        n207 = local read "Vdc_bias"() -> (w236:dbl)
        n208 = local read "Pdc SC"() -> (w256:dbl)
        n209 = local read "Vdc SC"() -> (w257:dbl)
        n210 = Add(x=w257, y=w236) -> (x+y=w237:dbl)
        n211 = local write "Start forming SC"(FALSE ("SEND sp")) -> ()
        n212 = call "Pdc_lim.vi"("IN Vdc"=w256) -> ("OUT Vdc"=w241:dbl)  [unwired: 10 in]
        n213 = call "V_limiter.vi"("IN Q"=w237) -> ("OUT Q"=w251:dbl)  [unwired: 10 in]
        n214 = To Word Integer(number=w241) -> (16bit integer=w245:i16)
        n215 = To Unsigned Word Integer(number=w251) -> (unsigned 16bit integer=w252:u16)
        n216 = Split Number(x=u16 4) -> (hi(x)=w247:u8, lo(x)=w248:u8)
        n217 = Split Number(x=w245) -> (hi(x)=w250:u8, lo(x)=w249:u8)
        n218 = Split Number(x=w252) -> (hi(x)=w254:u8, lo(x)=w253:u8)
        n219 = Split Number(x=u16 0 ("element")) -> (hi(x)=w242:u8, lo(x)=w243:u8)
        n220 = Build Array(w248, w247, w249, w250, w253, w254, w242, w243) -> (w240:u8[])
        n221 = flat-sequence {
          tunnel: [w259] -> w258
          tunnel: [w263] -> w238
          tunnel: w258 -> [w263]
          frame #0 {
            n222 = local read "Ready SC"() -> (w261:bool)
            n223 = local read "ON SC"() -> (w260:bool)
            n224 = Or(x=w260, y=w261) -> (x .or. y?=w259:bool)
          }
          frame #1 {
            n225 = Wait (ms)(milliseconds to wait=u32 20) -> ()  [unwired: 1 out]
          }
        }
      }
      frame 3 {
        # "it take on average 140ms to open the switch\n-> to be sure the grid is connected before we stors following, we add a 300ms delay\n-> the converter can easily sustain 160ms in forming mode when grid connected"
        # "SC"
        # "0x00C"
        # "send sp"
        n226 = local read "Vdc_bias"() -> (w264:dbl)
        n227 = local read "Pdc SC"() -> (w284:dbl)
        n228 = local read "Vdc SC"() -> (w285:dbl)
        n229 = Add(x=w285, y=w264) -> (x+y=w265:dbl)
        n230 = local write "Start following SC"(FALSE ("SEND sp")) -> ()
        n231 = call "Pdc_lim.vi"("IN Vdc"=w284) -> ("OUT Vdc"=w269:dbl)  [unwired: 10 in]
        n232 = call "V_limiter.vi"("IN Q"=w265) -> ("OUT Q"=w279:dbl)  [unwired: 10 in]
        n233 = To Word Integer(number=w269) -> (16bit integer=w273:i16)
        n234 = To Unsigned Word Integer(number=w279) -> (unsigned 16bit integer=w280:u16)
        n235 = Split Number(x=u16 3) -> (hi(x)=w275:u8, lo(x)=w276:u8)
        n236 = Split Number(x=w273) -> (hi(x)=w278:u8, lo(x)=w277:u8)
        n237 = Split Number(x=w280) -> (hi(x)=w282:u8, lo(x)=w281:u8)
        n238 = Split Number(x=u16 0 ("element")) -> (hi(x)=w270:u8, lo(x)=w271:u8)
        n239 = Build Array(w276, w275, w277, w278, w281, w282, w270, w271) -> (w266:u8[])
        n240 = local read "Ready SC"() -> (w286:bool)
        n241 = local read "ON SC"() -> (w287:bool)
        n242 = Or(x=w287, y=w286) -> (x .or. y?=w268:bool)
      }
      frame 100, Default {
      }
    }
    n243 = Get Date/Time In Seconds() -> (seconds since 1Jan1904=w157:timestamp)
    n244 = Get Date/Time In Seconds() -> (seconds since 1Jan1904=w145:timestamp)
    n245 = Bundle By Name(cluster=T1 {"timestamp"=timestamp(0 s since 1904-01-01), "payload"=[], "identifier"=0, "type"=0, "extended?"=FALSE, "echo?"=FALSE} ("CAN frame 3"), "payload"=w158, "identifier"=w193, "timestamp"=w157) -> (w190:T1)
    n246 = Bundle By Name(cluster=T1 {"timestamp"=timestamp(0 s since 1904-01-01), "payload"=[], "identifier"=0, "type"=0, "extended?"=FALSE, "echo?"=FALSE} ("CAN frame 3"), "payload"=w143, "identifier"=w142, "timestamp"=w145) -> (w146:T1)
    n247 = case shown="True" w191 {
      tunnel: w190 -> [w292 _]
      tunnel: w189 -> [w294 _]
      tunnel: [w293 _] -> w188
      frame True {
        n248 = Build Array(w292) -> (w295:T1[])
        n249 = call-poly <vilib>:"XNET Write.vi"("session in"=w294, "data"=w295) -> ("session out"=w293:refnum<k21>)  [unwired: 12 in, 1 out]
        "CAN OUT" <- w292
      }
      frame False {
      }
    }
    n250 = case shown="True" w141 {
      tunnel: w146 -> [w194 _]
      tunnel: w140 -> [w196 _]
      tunnel: [w195 _] -> w144
      frame True {
        n251 = Build Array(w194) -> (w197:T1[])
        n252 = call-poly <vilib>:"XNET Write.vi"("session in"=w196, "data"=w197) -> ("session out"=w195:refnum<k21>)  [unwired: 12 in, 1 out]
        "CAN OUT 2" <- w194
      }
      frame False {
      }
    }
    n253 = local read "main stop"() -> (w187:bool)
    n254 = node-c288() -> ()  [unwired: 1 in, 1 out]
  }
  n255 = timed-loop {
    timing: w89 -> [_]
    timing-out: [_] -> w88
    tunnel: w11 -> [w596]
    tunnel: [w600] -> w92
    tunnel: [FALSE ("stop CAN")] -> w90
    shift-right: [w594] -> _
    shift-left: T5 {"V_PV1"=0.0, "V_CAP1"=0.0, "V_PV2"=0.0, "V_CAP2"=0.0, "V_grid2"=0.0, "V_PV3"=0.0, "V_CAP3"=0.0, "V_grid3"=0.0, "V_PV4"=0.0, "V_CAP4"=0.0, "V_grid4"=0.0, "V_grid1"=0.0, "P1"=0.0, "P2"=0.0, "P3"=0.0, "P4"=0.0} ("measurements 2") -> [w595]
    shift-right: [w591] -> _
    shift-left: T4 {"V_SC"=0.0, "V_CAP"=0.0, "V_grid"=0.0, "P"=0.0, "SOC"=0.0} ("measurements SuperCap") -> [w592]
    tunnel: [w590] -> w14
    tunnel: w10 -> [w589]
    tunnel: w12 -> [w586]
    tunnel: w12 -> [w585]
    stop <- w599 stop-if-true
    # "READ CAN FROM CONVERTER"
    n256 = node-c288() -> ()  [unwired: 1 in, 1 out]
    n257 = Get Date/Time In Seconds() -> (seconds since 1Jan1904=→"current time":timestamp)
    n258 = local write "CAN with Conv"(TRUE) -> ()
    n259 = call-poly <vilib>:"XNET Read.vi"("session in"=w596, "error in (no error)"=w586) -> ("session out"=w600:refnum<k21>, "data"=w588:T1[])  [unwired: 10 in, 2 out]
    n260 = call-poly <vilib>:"XNET Read.vi"("session in"=w589, "error in (no error)"=w585) -> ("session out"=w590:refnum<k21>, "data"=w587:T1[])  [unwired: 10 in, 2 out]
    n261 = for {
      tunnel: w588 -> [w650] mode=indexing
      shift-right: [w648] -> w594
      shift-left: w595 -> [w649]
      n262 = Unbundle By Name(w650) -> ("payload"=w647:u8[], "identifier"=w646:u32)
      n263 = case shown="5" w646 {
        tunnel: w647 -> [_ w657 w663 w669 w675 w678 w704 w730 w756]
        tunnel: w649 -> [w651 w655 w661 w667 w673 w679 w705 w731 w757]
        tunnel: [w651 w656 w662 w668 w674 w680 w706 w732 w758] -> w648
        frame 0, Default {
        }
        frame 1 {
          # "0x001"
          # "P"
          n264 = call "U8arrayToMeasurement.vi"("payload"=w657) -> ("Meas 4"=w652:dbl, "Meas 1"=w653:dbl, "Meas 2"=w654:dbl)  [unwired: 4 in, 1 out]
          "V slider 28" <- w653
          "V slider 27" <- w652
          n265 = Bundle By Name(cluster=w655, "V_CAP1"=w654, "V_PV1"=w653, "V_grid1"=w652) -> (w656:T5)
        }
        frame 4 {
          # "0x004"
          # "P"
          n266 = call "U8arrayToMeasurement.vi"("payload"=w663) -> ("Meas 4"=w658:dbl, "Meas 1"=w659:dbl, "Meas 2"=w660:dbl)  [unwired: 4 in, 1 out]
          "V slider 26" <- w659
          "V slider 25" <- w658
          n267 = Bundle By Name(cluster=w661, "V_CAP2"=w660, "V_PV2"=w659, "V_grid2"=w658) -> (w662:T5)
        }
        frame 7 {
          # "0x007"
          # "P"
          n268 = call "U8arrayToMeasurement.vi"("payload"=w669) -> ("Meas 4"=w664:dbl, "Meas 1"=w665:dbl, "Meas 2"=w666:dbl)  [unwired: 4 in, 1 out]
          "V slider 24" <- w665
          "V slider 23" <- w664
          n269 = Bundle By Name(cluster=w667, "V_CAP3"=w666, "V_PV3"=w665, "V_grid3"=w664) -> (w668:T5)
        }
        frame 10 {
          # "0x00A"
          # "P"
          n270 = call "U8arrayToMeasurement.vi"("payload"=w675) -> ("Meas 4"=w671:dbl, "Meas 1"=w670:dbl, "Meas 2"=w672:dbl)  [unwired: 4 in, 1 out]
          "V slider 21" <- w671
          "V slider 22" <- w670
          n271 = Bundle By Name(cluster=w673, "V_CAP4"=w672, "V_PV4"=w670, "V_grid4"=w671) -> (w674:T5)
        }
        frame 2 {
          # "0x002"
          n272 = call "U8arrayToMeasurement2.vi"("payload"=w678) -> ("Meas 2"=w676:dbl, "uint16"=w677:u16)  [unwired: 4 in, 2 out]
          "kW" <- w676
          "state 1" <- w677
          n273 = case shown="1" w677 {
            frame 3 {
              # "idle"
              n274 = local write "ON 1"(FALSE ("ON 1")) -> ()
              n275 = local write "Ready 1"(TRUE ("Ready 1")) -> ()
              n276 = local write "OFF 1"(FALSE ("OFF 1")) -> ()
            }
            frame 4 {
              # "mppt"
              n277 = local write "ON 1"(FALSE ("ON 1")) -> ()
              n278 = local write "Ready 1"(TRUE ("Ready 1")) -> ()
              n279 = local write "OFF 1"(FALSE ("OFF 1")) -> ()
            }
            frame 5 {
              # "mppt"
              n280 = local write "ON 1"(TRUE ("ON 1")) -> ()
              n281 = local write "Ready 1"(FALSE ("Ready 1")) -> ()
              n282 = local write "OFF 1"(FALSE ("OFF 1")) -> ()
            }
            frame 0 {
              # "to precharge"
              n283 = local write "ON 1"(FALSE ("ON 1")) -> ()
              n284 = local write "Ready 1"(FALSE ("Ready 1")) -> ()
              n285 = local write "OFF 1"(TRUE ("OFF 1")) -> ()
            }
            frame 6, Default {
              # "to precharge"
              n286 = local write "ON 1"(FALSE ("ON 1")) -> ()
              n287 = local write "Ready 1"(FALSE ("Ready 1")) -> ()
              n288 = local write "OFF 1"(FALSE ("OFF 1")) -> ()
            }
            frame 1 {
              # "precharge"
              n289 = local write "ON 1"(FALSE ("ON 1")) -> ()
              n290 = local write "Ready 1"(FALSE ("Ready 1")) -> ()
              n291 = local write "OFF 1"(TRUE ("OFF 1")) -> ()
            }
            frame 2 {
              # "standby"
              n292 = local write "ON 1"(FALSE ("ON 1")) -> ()
              n293 = local write "Ready 1"(TRUE ("Ready 1")) -> ()
              n294 = local write "OFF 1"(FALSE ("OFF 1")) -> ()
            }
          }
          n295 = Bundle By Name(cluster=w679, "P1"=w676) -> (w680:T5)
        }
        frame 5 {
          # "0x005"
          n296 = call "U8arrayToMeasurement2.vi"("payload"=w704) -> ("Meas 2"=w702:dbl, "uint16"=w703:u16)  [unwired: 4 in, 2 out]
          "state 2" <- w703
          "kW" <- w702
          n297 = case shown="6, Default" w703 {
            frame 3 {
              # "idle"
              n298 = local write "ON 2"(FALSE ("ON 1")) -> ()
              n299 = local write "Ready 2"(TRUE ("Ready 1")) -> ()
              n300 = local write "OFF 2"(FALSE ("OFF 1")) -> ()
            }
            frame 4 {
              # "mppt"
              n301 = local write "ON 2"(FALSE ("ON 1")) -> ()
              n302 = local write "Ready 2"(TRUE ("Ready 1")) -> ()
              n303 = local write "OFF 2"(FALSE ("OFF 1")) -> ()
            }
            frame 5 {
              # "mppt"
              n304 = local write "ON 2"(TRUE ("ON 1")) -> ()
              n305 = local write "Ready 2"(FALSE ("Ready 1")) -> ()
              n306 = local write "OFF 2"(FALSE ("OFF 1")) -> ()
            }
            frame 0 {
              # "to precharge"
              n307 = local write "ON 2"(FALSE ("ON 1")) -> ()
              n308 = local write "Ready 2"(FALSE ("Ready 1")) -> ()
              n309 = local write "OFF 2"(TRUE ("OFF 1")) -> ()
            }
            frame 6, Default {
              # "to precharge"
              n310 = local write "ON 2"(FALSE ("ON 1")) -> ()
              n311 = local write "Ready 2"(FALSE ("Ready 1")) -> ()
              n312 = local write "OFF 2"(FALSE ("OFF 1")) -> ()
            }
            frame 1 {
              # "precharge"
              n313 = local write "ON 2"(FALSE ("ON 1")) -> ()
              n314 = local write "Ready 2"(FALSE ("Ready 1")) -> ()
              n315 = local write "OFF 2"(TRUE ("OFF 1")) -> ()
            }
            frame 2 {
              # "standby"
              n316 = local write "ON 2"(FALSE ("ON 1")) -> ()
              n317 = local write "Ready 2"(TRUE ("Ready 1")) -> ()
              n318 = local write "OFF 2"(FALSE ("OFF 1")) -> ()
            }
          }
          n319 = Bundle By Name(cluster=w705, "P2"=w702) -> (w706:T5)
        }
        frame 8 {
          # "0x008"
          n320 = call "U8arrayToMeasurement2.vi"("payload"=w730) -> ("Meas 2"=w728:dbl, "uint16"=w729:u16)  [unwired: 4 in, 2 out]
          "state 3" <- w729
          "kW" <- w728
          n321 = case shown="2" w729 {
            frame 3 {
              # "idle"
              n322 = local write "ON 3"(FALSE ("ON 1")) -> ()
              n323 = local write "Ready 3"(TRUE ("Ready 1")) -> ()
              n324 = local write "OFF 3"(FALSE ("OFF 1")) -> ()
            }
            frame 4 {
              # "mppt"
              n325 = local write "ON 3"(FALSE ("ON 1")) -> ()
              n326 = local write "Ready 3"(TRUE ("Ready 1")) -> ()
              n327 = local write "OFF 3"(FALSE ("OFF 1")) -> ()
            }
            frame 5 {
              # "mppt"
              n328 = local write "ON 3"(TRUE ("ON 1")) -> ()
              n329 = local write "Ready 3"(FALSE ("Ready 1")) -> ()
              n330 = local write "OFF 3"(FALSE ("OFF 1")) -> ()
            }
            frame 0 {
              # "to precharge"
              n331 = local write "ON 3"(FALSE ("ON 1")) -> ()
              n332 = local write "Ready 3"(FALSE ("Ready 1")) -> ()
              n333 = local write "OFF 3"(TRUE ("OFF 1")) -> ()
            }
            frame 6, Default {
              # "to precharge"
              n334 = local write "ON 3"(FALSE ("ON 1")) -> ()
              n335 = local write "Ready 3"(FALSE ("Ready 1")) -> ()
              n336 = local write "OFF 3"(FALSE ("OFF 1")) -> ()
            }
            frame 1 {
              # "precharge"
              n337 = local write "ON 3"(FALSE ("ON 1")) -> ()
              n338 = local write "Ready 3"(FALSE ("Ready 1")) -> ()
              n339 = local write "OFF 3"(TRUE ("OFF 1")) -> ()
            }
            frame 2 {
              # "standby"
              n340 = local write "ON 3"(FALSE ("ON 1")) -> ()
              n341 = local write "Ready 3"(TRUE ("Ready 1")) -> ()
              n342 = local write "OFF 3"(FALSE ("OFF 1")) -> ()
            }
          }
          n343 = Bundle By Name(cluster=w731, "P3"=w728) -> (w732:T5)
        }
        frame 11 {
          # "0x00B"
          n344 = call "U8arrayToMeasurement2.vi"("payload"=w756) -> ("Meas 2"=w754:dbl, "uint16"=w755:u16)  [unwired: 4 in, 2 out]
          "state 4" <- w755
          "kW" <- w754
          n345 = case shown="5" w755 {
            frame 3 {
              # "idle"
              n346 = local write "ON 4"(FALSE ("ON 1")) -> ()
              n347 = local write "Ready 4"(TRUE ("Ready 1")) -> ()
              n348 = local write "OFF 4"(FALSE ("OFF 1")) -> ()
            }
            frame 4 {
              # "mppt"
              n349 = local write "ON 4"(FALSE ("ON 1")) -> ()
              n350 = local write "Ready 4"(TRUE ("Ready 1")) -> ()
              n351 = local write "OFF 4"(FALSE ("OFF 1")) -> ()
            }
            frame 5 {
              # "mppt"
              n352 = local write "ON 4"(TRUE ("ON 1")) -> ()
              n353 = local write "Ready 4"(FALSE ("Ready 1")) -> ()
              n354 = local write "OFF 4"(FALSE ("OFF 1")) -> ()
            }
            frame 0 {
              # "to precharge"
              n355 = local write "ON 4"(FALSE ("ON 1")) -> ()
              n356 = local write "Ready 4"(FALSE ("Ready 1")) -> ()
              n357 = local write "OFF 4"(TRUE ("OFF 1")) -> ()
            }
            frame 6, Default {
              # "to precharge"
              n358 = local write "ON 4"(FALSE ("ON 1")) -> ()
              n359 = local write "Ready 4"(FALSE ("Ready 1")) -> ()
              n360 = local write "OFF 4"(FALSE ("OFF 1")) -> ()
            }
            frame 1 {
              # "precharge"
              n361 = local write "ON 4"(FALSE ("ON 1")) -> ()
              n362 = local write "Ready 4"(FALSE ("Ready 1")) -> ()
              n363 = local write "OFF 4"(TRUE ("OFF 1")) -> ()
            }
            frame 2 {
              # "standby"
              n364 = local write "ON 4"(FALSE ("ON 1")) -> ()
              n365 = local write "Ready 4"(TRUE ("Ready 1")) -> ()
              n366 = local write "OFF 4"(FALSE ("OFF 1")) -> ()
            }
          }
          n367 = Bundle By Name(cluster=w757, "P4"=w754) -> (w758:T5)
        }
      }
      n368 = local write "measurements"(w648) -> ()
      "CAN IN" <- w650
    }
    n369 = for {
      shift-right: [w604] -> w591
      shift-left: w592 -> [w605]
      tunnel: w587 -> [w603] mode=indexing
      n370 = Unbundle By Name(w603) -> ("payload"=w602:u8[], "identifier"=w601:u32)
      n371 = case shown="E" w601 {
        tunnel: w602 -> [w608 _ w624]
        tunnel: w605 -> [w607 w620 w626]
        tunnel: [w606 w620 w625] -> w604
        frame 15 {
          # "0x00F"
          n372 = call "U8arrayToMeasurement2.vi"("payload"=w608) -> ("Meas 2"=w609:dbl, "uint16"=w612:u16)  [unwired: 4 in, 2 out]
          "state SC" <- w612
          "kW" <- w609
          n373 = Equal?(x=w612, y=u16 43) -> (x = y?=w615:bool)
          n374 = Equal?(x=w612, y=u16 44) -> (x = y?=w619:bool)
          "forming?" <- w619
          n375 = Equal?(x=w612, y=u16 41) -> (x = y?=w616:bool)
          n376 = Or(x=w615, y=w619) -> (x .or. y?=w610:bool)
          n377 = Compound Arithmetic op=OR(w615, w619, w616) -> (w617:bool)
          n378 = local write "Ready SC"(w616) -> ()
          n379 = Bundle By Name(cluster=w607, "P"=w609) -> (w606:T4)
          n380 = Not(x=w617) -> (.not. x?=w618:bool)
          n381 = local write "ON SC"(w610) -> ()
          n382 = local write "OFF SC"(w618) -> ()
        }
        frame 0, Default {
        }
        frame 14 {
          w635 = i16 -2 ("n")
          w636 = 16.0 ("Meas 1")
          # "Vmax"
          # "Vmin"
          # "F"
          # "0x00E"
          # "P"
          n383 = call "U8arrayToMeasurement.vi"("payload"=w624) -> ("Meas 4"=w645:dbl, "Meas 1"=w622:dbl, "Meas 2"=w623:dbl)  [unwired: 4 in, 1 out]
          "V slider 30" <- w622
          "V slider 29" <- w623
          n384 = Square(x=150.0 ("Meas 1")) -> (x^2=w641:dbl)
          n385 = Square(x=300.0 ("Meas 1")) -> (x^2=w642:dbl)
          n386 = Square(x=w622) -> (x^2=w638:dbl)
          n387 = Multiply(x=w641, y=w636) -> (x*y=w640:dbl)
          n388 = Multiply(x=w642, y=w636) -> (x*y=w639:dbl)
          n389 = Multiply(x=w638, y=w636) -> (x*y=w637:dbl)
          n390 = Scale By Power Of 2(n=w635, x=w640) -> (x*2^n=w632:dbl)
          n391 = Scale By Power Of 2(n=w635, x=w637) -> (x*2^n=w634:dbl)
          n392 = Scale By Power Of 2(n=w635, x=w639) -> (x*2^n=w633:dbl)
          n393 = Subtract(x=w634, y=w632) -> (x-y=w631:dbl)
          n394 = Subtract(x=w633, y=w632) -> (x-y=w630:dbl)
          n395 = Divide(x=w631, y=w630) -> (x/y=w629:dbl)
          n396 = Multiply(x=w629, y=100.0) -> (x*y=w628:dbl)
          n397 = Round To Nearest(number=w628) -> (nearest integer value=w621:dbl)
          "V slider 31" <- w621
          n398 = Bundle By Name(cluster=w626, "V_CAP"=w623, "V_SC"=w622, "V_grid"=w645, "SOC"=w621) -> (w625:T4)
        }
      }
      n399 = local write "measurements SuperCap"(w604) -> ()
      "CAN frame" <- w603
    }
    n400 = local read "main stop"() -> (w599:bool)
    n401 = node-c288() -> ()  [unwired: 1 in, 1 out]
  }
  n402 = String To IP(1:w83) -> (0:w23:u32)
  n403 = while {
    tunnel: w38 -> [w786]
    tunnel: [w787] -> w33
    shift-right: [w788] -> _
    shift-left: T3 {"Synchronized?"=FALSE, "Sync Loss Count in"=0, "Current Sync Duration"=0} ("Status In") -> [w789]
    tunnel: w36 -> [w790]
    tunnel: "Loop Time" -> [w783]
    tunnel: [w785] -> w34
    stop <- w782 stop-if-true
    # "Run in parallel with \nyour other loops"
    # "Check Time Synch"
    n404 = Wait (ms)(milliseconds to wait=w783) -> ()  [unwired: 1 out]
    n405 = call "PM_Synch_Monitor.vi"("Polling Interval"=w783, "error in"=w786, "Status In"=w789, "Synch In"=w790) -> ("error out"=w787:errorcluster, "Status Out"=w788:T3, "Reference out"=w785:refnum<k15>, "Offset from TR (ns)"=→"Offset from TR (ns)":dbl)  [unwired: 3 in, 1 out]
    "Status Out" <- w788
    n406 = local read "main stop"() -> (w782:bool)
  }
  n407 = UDP Open(11:w84) -> (port=w21:refnum<k16>, 0:w20:errorcluster)  [unwired: 4 in, 1 out]
  n408 = while {
    tunnel: [w799] -> w24
    tunnel: w23 -> [w798]
    tunnel: w22 -> [w797]
    tunnel: w20 -> [w795]
    shift-right: [w794] -> w19
    shift-left: w21 -> [w796]
    stop <- w793 stop-if-true
    n409 = local read "measurements"() -> (w807:T5)
    n410 = local read "measurements SuperCap"() -> (w813:T4)
    n411 = Get Date/Time In Seconds() -> (seconds since 1Jan1904=w802:timestamp)
    n412 = To Double Precision Float(number=w802) -> (double precision float=w806:dbl)
    n413 = local read "ON SC"() -> (w814:bool)
    n414 = Wait Until Next ms Multiple(millisecond multiple=u32 100) -> ()  [unwired: 1 out]
    n415 = local read "ON 1"() -> (w808:bool)
    n416 = local read "ON 2"() -> (w809:bool)
    n417 = local read "ON 3"() -> (w810:bool)
    n418 = local read "ON 4"() -> (w811:bool)
    n419 = Bundle By Name(cluster=T13 {"Info"={"Resource"="PV_emulator", "Problem"=FALSE, "Timestamp"=0.0}, "Data"={"Status 1"=FALSE, "Status 2"=FALSE, "measurements"={"V_PV1"=0.0, "V_CAP1"=0.0, "V_PV2"=0.0, "V_CAP2"=0.0, "V_grid2"=0.0, "V_PV3"=0.0, "V_CAP3"=0.0, "V_grid3"=0.0, "V_PV4"=0.0, "V_CAP4"=0.0, "V_grid4"=0.0, "V_grid1"=0.0, "P1"=0.0, "P2"=0.0, "P3"=0.0, "P4"=0.0}, "Status 3"=FALSE, "Status 4"=FALSE, "measurements SC"={"V_SC"=0.0, "V_CAP"=0.0, "V_grid"=0.0, "P"=0.0, "SOC"=0.0}, "Status SC"=FALSE, "Forming/Following"=FALSE, "Start forming"=FALSE, "SC references"={"Vdc"=0.0, "Pdc"=0.0}, "Start following"=FALSE}} ("Cluster"), "Info.Resource"="PV_emulator", "Info.Problem"=FALSE, "Info.Timestamp"=w806, "Data.Status 1"=w808, "Data.Status 2"=w809, "Data.Status 3"=w810, "Data.Status 4"=w811, "Data.Status SC"=w814, "Data.measurements"=w807, "Data.measurements SC"=w813) -> (w812:T13)
    n420 = Flatten To JSON(anything=w812, error in (no error)=w795) -> (JSON string=w801:string, 11:w800:errorcluster)  [unwired: 1 in]
    n421 = UDP Write(address=w798, port or service name=w797, connection ID=w796, data in=w801, 8:w800, 9:50 ("timeout ms (25000)")) -> (error out=w816:errorcluster, 3:w794:refnum<k16>)
    n422 = local read "main stop"() -> (w793:bool)
    n423 = call <vilib>:"Clear Errors.vi"("error in (no error)"=w816, "specific error code to clear (0: all)"=56) -> ("error out"=w799:errorcluster)  [unwired: 4 in, 1 out]
  }
  n424 = String To IP(1:w29) -> (0:w30:u32)
  n425 = UDP Open(7:w30, 11:w28) -> (port=w26:refnum<k16>, 0:w27:errorcluster)  [unwired: 3 in, 1 out]
  n426 = node-c288(w81) -> ()  [unwired: 1 out]
  n427 = UDP Close(connection ID=w41, 8:w40) -> ()  [unwired: 2 out]
  n428 = while {
    tunnel: w27 -> [w820]
    shift-right: [w830] -> w25
    shift-left: w26 -> [w821]
    tunnel: [w828] -> w17
    stop <- w832 stop-if-true
    # "Clear errors due\nto timeout"
    # "UDP stream"
    n429 = UDP Read(connection ID=w821, max size (548)=1000, timeout ms (25000)=50, 8:w820) -> (data out=w825:string, error out=w827:errorcluster, 3:w830:refnum<k16>)  [unwired: 2 out]
    n430 = Wait Until Next ms Multiple(millisecond multiple=u32 100) -> ()  [unwired: 1 out]
    n431 = Unflatten From JSON(JSON string=w825, type and defaults=T13 {"Info"={"Resource"="PV_emulator", "Problem"=FALSE, "Timestamp"=0.0}, "Data"={"Status 1"=FALSE, "Status 2"=FALSE, "measurements"={"V_PV1"=0.0, "V_CAP1"=0.0, "V_PV2"=0.0, "V_CAP2"=0.0, "V_grid2"=0.0, "V_PV3"=0.0, "V_CAP3"=0.0, "V_grid3"=0.0, "V_PV4"=0.0, "V_CAP4"=0.0, "V_grid4"=0.0, "V_grid1"=0.0, "P1"=0.0, "P2"=0.0, "P3"=0.0, "P4"=0.0}, "Status 3"=FALSE, "Status 4"=FALSE, "measurements SC"={"V_SC"=0.0, "V_CAP"=0.0, "V_grid"=0.0, "P"=0.0, "SOC"=0.0}, "Status SC"=FALSE, "Forming/Following"=FALSE, "Start forming"=FALSE, "SC references"={"Vdc"=0.0, "Pdc"=0.0}, "Start following"=FALSE}} ("Cluster"), error in (no error)=w827) -> (value=w823:T13, error out=w826:errorcluster)  [unwired: 4 in]
    n432 = Unbundle By Name(w823) -> ("Data.Start forming"=w817:bool, "Data.Start following"=w818:bool, "Data.SC references"=w822:T16)
    n433 = case shown="No Error" w826 {
      selector: w826 -> [w840 w904]
      tunnel: [w845 w904] -> w828
      tunnel: w822 -> [w836 _]
      tunnel: w822 -> [w835 _]
      tunnel: w818 -> [w834 _]
      tunnel: w817 -> [w833 _]
      frame No Error {
        n434 = local write "Start forming SC"(w833) -> ()
        n435 = disable-structure shown="Disabled" {
          disable-tunnel: [w884 _] -> w844
          disable-tunnel: w840 -> [w883 _]
          disable-tunnel: w835 -> [w882 _]
          frame Disabled {
            n436 = flat-sequence {
              tunnel: w883 -> [w891]
              tunnel: [w891] -> w886
              tunnel: [w890] -> w885
              tunnel: w882 -> [w889]
              tunnel: w886 -> [w893]
              tunnel: [w893] -> w884
              tunnel: w885 -> [w892]
              frame #0 {
                n437 = local read "ON 1"() -> (w890:bool)
                n438 = Unbundle(w889) -> ()  [unwired: 2 out]
                n439 = call "Q_limiter.vi"("IN Q"=0.0) -> ("OUT Q"=w888:dbl)  [unwired: 10 in]
                n440 = local write "P 1"(w888) -> ()
              }
              frame #1 {
                n441 = local write "PowerEnable 1"(w892) -> ()
              }
            }
          }
          frame Enabled {
          }
        }
        n442 = disable-structure shown="Disabled" {
          disable-tunnel: [w872 _] -> w842
          disable-tunnel: w840 -> [w871 _]
          disable-tunnel: w835 -> [w870 _]
          frame Disabled {
            n443 = flat-sequence {
              tunnel: w871 -> [w879]
              tunnel: w870 -> [w878]
              tunnel: [w879] -> w874
              tunnel: [w877] -> w873
              tunnel: [w881] -> w872
              tunnel: w874 -> [w881]
              tunnel: w873 -> [w880]
              frame #0 {
                n444 = local read "ON 2"() -> (w877:bool)
                n445 = Unbundle(w878) -> ()  [unwired: 2 out]
                n446 = call "Q_limiter.vi"("IN Q"=0.0) -> ("OUT Q"=w876:dbl)  [unwired: 10 in]
                n447 = local write "P 2"(w876) -> ()
              }
              frame #1 {
                n448 = local write "PowerEnable 2"(w880) -> ()
              }
            }
          }
          frame Enabled {
          }
        }
        n449 = disable-structure shown="Disabled" {
          disable-tunnel: [w860 _] -> w843
          disable-tunnel: w840 -> [w859 _]
          disable-tunnel: w835 -> [w858 _]
          frame Disabled {
            n450 = flat-sequence {
              tunnel: w859 -> [w867]
              tunnel: w858 -> [w866]
              tunnel: [w867] -> w862
              tunnel: [w865] -> w861
              tunnel: [w869] -> w860
              tunnel: w862 -> [w869]
              tunnel: w861 -> [w868]
              frame #0 {
                n451 = local read "ON 3"() -> (w865:bool)
                n452 = Unbundle(w866) -> ()  [unwired: 2 out]
                n453 = call "Q_limiter.vi"("IN Q"=0.0) -> ("OUT Q"=w864:dbl)  [unwired: 10 in]
                n454 = local write "P 3"(w864) -> ()
              }
              frame #1 {
                n455 = local write "PowerEnable 3"(w868) -> ()
              }
            }
          }
          frame Enabled {
          }
        }
        n456 = disable-structure shown="Disabled" {
          disable-tunnel: w840 -> [w848 _]
          disable-tunnel: [w847 _] -> w838
          disable-tunnel: w835 -> [w846 _]
          frame Disabled {
            n457 = flat-sequence {
              tunnel: w848 -> [w855]
              tunnel: [w854] -> _
              tunnel: w846 -> [w854]
              tunnel: [w855] -> w850
              tunnel: [w853] -> w849
              tunnel: [w857] -> w847
              tunnel: w850 -> [w857]
              tunnel: w849 -> [w856]
              frame #0 {
                n458 = local read "ON 4"() -> (w853:bool)
                n459 = Unbundle(w854) -> ()  [unwired: 2 out]
                n460 = call "Q_limiter.vi"("IN Q"=0.0) -> ("OUT Q"=w852:dbl)  [unwired: 10 in]
                n461 = local write "P 4"(w852) -> ()
              }
              frame #1 {
                n462 = local write "PowerEnable 4"(w856) -> ()
              }
            }
          }
          frame Enabled {
          }
        }
        n463 = flat-sequence {
          tunnel: [w894] -> w841
          tunnel: w840 -> [w898]
          tunnel: [w898] -> w839
          tunnel: w836 -> [w899]
          tunnel: w841 -> [w903]
          tunnel: [w902] -> w837
          tunnel: w839 -> [w902]
          frame #0 {
            n464 = local read "ON SC"() -> (w894:bool)
            n465 = Unbundle By Name(w899) -> ("Vdc"=w901:dbl, "Pdc"=w900:dbl)
            n466 = call "V_limiter.vi"("IN Q"=w901) -> ("OUT Q"=w895:dbl)  [unwired: 10 in]
            n467 = call "Q_limiter.vi"("IN Q"=w900) -> ("OUT Q"=w897:dbl)  [unwired: 10 in]
            n468 = Round To Nearest(number=w897) -> (nearest integer value=w896:dbl)
            n469 = local write "Vdc SC"(w895) -> ()
            n470 = local write "Pdc SC"(w896) -> ()
          }
          frame #1 {
            n471 = local write "SEND sp SC"(w903) -> ()
          }
        }
        n472 = Merge Errors(w844, w842, w843, w838, w837) -> (w845:errorcluster)
        "start following SC pre" <- w834
      }
      frame Error {
      }
    }
    n473 = local read "main stop"() -> (w832:bool)
  }
  n474 = TCP Close Connection(connection ID=w73, error in (no error)=w72) -> (error out=w74:errorcluster)  [unwired: 1 in, 1 out]
  n475 = TCP Close Connection(connection ID=w49, error in (no error)=w48) -> (error out=w52:errorcluster)  [unwired: 1 in, 1 out]
  n476 = TCP Close Connection(connection ID=w47, error in (no error)=w46) -> (error out=w51:errorcluster)  [unwired: 1 in, 1 out]
  n477 = TCP Close Connection(connection ID=w45, error in (no error)=w44) -> (error out=w50:errorcluster)  [unwired: 1 in, 1 out]
  n478 = call <vilib>:"General Error Handler.vi"("error in (no error)"=w74) -> ()  [unwired: 10 in, 5 out]
  n479 = call <vilib>:"General Error Handler.vi"("error in (no error)"=w52) -> ()  [unwired: 10 in, 5 out]
  n480 = call <vilib>:"General Error Handler.vi"("error in (no error)"=w51) -> ()  [unwired: 10 in, 5 out]
  n481 = call <vilib>:"General Error Handler.vi"("error in (no error)"=w50) -> ()  [unwired: 10 in, 5 out]
  n482 = call <instrlib>:"niSync Close.vi"("error in (no error)"=w33, "instrument handle"=w34) -> ("error out"=→"Error out":errorcluster)  [unwired: 9 in]
  n483 = while {
    stop <- w905 stop-if-true
    n484 = flat-sequence {
      tunnel: [w907] -> w906
      tunnel: w906 -> [w914]
      frame #0 {
        n485 = local read "start following SC pre"() -> (w908:bool)
        n486 = call <userlib>:"Boolean Trigger__ogtk.vi"("Boolean Input"=w908) -> ("Rising Edge"=w909:bool)  [unwired: 1 in, 1 out]
        n487 = case shown="True" w909 {
          tunnel: w908 -> [w910 w911]
          tunnel: [w910 w911] -> w907
          frame False {
          }
          frame True {
            # "650"
            n488 = Get Date/Time In Seconds() -> (seconds since 1Jan1904=→"time_sc":timestamp)
            n489 = Wait (ms)(milliseconds to wait=u32 650) -> ()  [unwired: 1 out]
          }
        }
      }
      frame #1 {
        n490 = local write "Start following SC"(w914) -> ()
      }
    }
    n491 = local read "main stop"() -> (w905:bool)
  }
  n492 = UDP Close(connection ID=w19, 8:w24) -> ()  [unwired: 2 out]
  n493 = node-c288(w88) -> ()  [unwired: 1 out]
  n494 = call <vilib>:"XNET Stop.vi"("session in"=w14) -> ()  [unwired: 13 in, 2 out]
  n495 = node-c288(i64 10 ("Period")) -> (w3:T7)  [unwired: 3 in]
  n496 = timed-loop {
    tunnel: 325 -> [w918]
    shift-right: [w924] -> _
    shift-left: dbl[] [] ("SOC") -> [w925]
    timing: w3 -> [_]
    timing-out: [_] -> w2
    stop <- w917 stop-if-true
    (unwired) i64 0 ("Iteration Duration")
    n497 = node-c288() -> (→"Finished Late? [i-1]":bool, →"Iteration Duration":i64)  [unwired: 1 in]
    n498 = local read "measurements SuperCap"() -> (w923:T4)
    n499 = Array Size(array=w925) -> (size(s)=w927:i32)
    n500 = Equal?(x=w927, y=w918) -> (x = y?=w926:bool)
    n501 = Unbundle By Name(w923) -> ("SOC"=w920:dbl)
    n502 = case shown="False" w926 {
      tunnel: w925 -> [w934 w942]
      tunnel: w920 -> [w933 w940]
      tunnel: [w932 w935] -> w924
      tunnel: w918 -> [_ w936]
      frame False {
        n503 = Insert Into Array(array=w934, new element=w933) -> (w932:dbl[])  [unwired: 1 in]
      }
      frame True {
        n504 = Array Subset(array=w942, index=0) -> (w941:dbl[])  [unwired: 1 in]
        n505 = Build Array (concatenate)(w940, w941) -> (w938:dbl[])
        n506 = Delete From Array(array=w938, length=1, index=w936) -> (array with subset deleted=w935:dbl[])  [unwired: 1 out]
      }
    }
    n507 = call-poly <vilib>:"Mean.vi"("X"=w924) -> ("mean"=w919:dbl)  [unwired: 1 out]
    n508 = Bundle By Name(cluster=w923, "SOC"=w919) -> (w922:T4)
    n509 = Bundle("SOC"=w920, "mean"=w919) -> (→"SOC_plot":cluster{"SOC":dbl, "mean":dbl})  [unwired: 1 in]
    n510 = local write "measurements SuperCap"(w922) -> ()
    n511 = local read "main stop"() -> (w917:bool)
    n512 = node-c288() -> ()  [unwired: 1 in, 1 out]
  }
  n513 = node-c288(w85) -> ()  [unwired: 1 out]
  n514 = call <vilib>:"XNET Stop.vi"("session in"=w13) -> ()  [unwired: 13 in, 2 out]
  n515 = call <vilib>:"XNET Stop.vi"("session in"=w91) -> ()  [unwired: 13 in, 2 out]
  n516 = local write "CAN with Conv"(w90) -> ()
  n517 = call <vilib>:"XNET Stop.vi"("session in"=w92) -> ()  [unwired: 13 in, 2 out]
  n518 = node-c288(w2) -> ()  [unwired: 1 out]
  n519 = UDP Close(connection ID=w25, 8:w17) -> ()  [unwired: 2 out]
  "Measurements" <- w16
  "CAN with Conv" <- w16
  "Ready 1" <- w16
  "OFF 1" <- w16
  "Ready 2" <- w16
  "ON 2" <- w16
  "OFF 2" <- w16
  "Ready 4" <- w16
  "ON 4" <- w16
  "OFF 4" <- w16
  "ON 3" <- w16
  "Ready 3" <- w16
  "OFF 3" <- w16
  "ON SC" <- w16
  "OFF SC" <- w16
  "Ready SC" <- w16
